vi "Temp - Create DAQ Tasks.vi"(8 "error in (no error)":errorcluster, 10 "DAQ Configuration":T18={"AI Configuration"=[], "AO Configuration"=[], "AI Buffer Size (S)"=10, "sample mode"=10178, "input terminal configuration"=-1, "output terminal configuration"=-1, "Channels: AO"={"AO amp (V)"=[0.1, 0.09, 0.08, 0.07, 0.06, 0.05, 0.04, 0.03], "AO DC (V)"=[0.0, 0.0, 0.0, 0.0, 0.0, 0.0, 0.0, 0.0], "AO f (Hz)"=[13.0, 13.0, 13.0, 13.0, 13.0, 13.0, 13.0, 13.0], "AO phi (°)"=[0.0, 0.0, 0.0, 0.0, 0.0, 0.0, 0.0, 0.0], "function"=[enum."Sine", enum."Sine", enum."Sine", enum."Sine", enum."Sine", enum."Sine", enum."Sine", enum."Sine"], "I+"=[]}, "Channels: Lockin"={"REF f (Hz)"=[0.4, 0.4], "REF phi (°)"=[0.0, 0.0]}, "sampling info"={"Fs"=0.0, "#s"=0.0}} {"Channels: Lockin"."REF phi (°)" format="%#_3g"; "Channels: AO"."AO f (Hz)" min=0.001 max=10000.0; "Channels: AO"."AO DC (V)" format="%.3p"; "Channels: AO"."AO amp (V)" format="%.3p"; "output terminal configuration" items=["Default"=-1, "RSE"=10083, "Differential"=10106, "Pseudodifferential"=12529]; "input terminal configuration" items=["default"=-1, "RSE"=10083, "NRSE"=10078, "Differential"=10106, "Pseudodifferential"=12529]; "sample mode" items=["Finite Samples"=10178, "Continuous Samples"=10123]}, 11 "LockinDAQ in":refnum<class "LockinDAQ.lvclass">) -> (0 "error out":errorcluster, 3 "LockinDAQ out":refnum<class "LockinDAQ.lvclass">)   [LabVIEW 2016, in "LockinDAQ.lvclass"]
uses:
  LockinDAQ.lvclass
  Typedefs/AI.config-array.ctl
  Typedefs/AI.config-cluster.ctl
  Typedefs/AI.coupling-enum.ctl
  Typedefs/446xAI-enum.ctl
  Typedefs/AO.config-array.ctl
  Typedefs/AO.config-cluster.ctl
  Typedefs/446xAO-enum.ctl
  Typedefs/AO-cluster.ctl
  Typedefs/AO_Amp-array.ctl
  Typedefs/AO_DC-array.ctl
  Typedefs/AO_f-array.ctl
  Typedefs/AO_phi-array.ctl
  Typedefs/Function-array.ctl
  Typedefs/Function-enum.ctl
  Typedefs/REF-cluster.ctl
  Typedefs/REF_f-array.ctl
  Typedefs/REF_phi-array.ctl
  LockinDAQ.lvclass/LockinDAQ.ctl
  <vilib>/DAQmx/write.llb/DAQmx Write (Analog 1D Wfm NChan NSamp).vi
  <vilib>/DAQmx/read.llb/DAQmx Read (Analog 1D Wfm NChan NSamp).vi
  <vilib>/DAQmx/create/channels.llb/DAQmx Create Channel (AO-Voltage-Basic).vi
  <vilib>/DAQmx/create/channels.llb/DAQmx Create Channel (AI-Voltage-Basic).vi
  <vilib>/DAQmx/configure/timing.llb/DAQmx Timing (Sample Clock).vi
  <vilib>/DAQmx/configure/trigger.llb/DAQmx Start Trigger (Digital Edge).vi
  <vilib>/DAQmx/miscellaneous.llb/DAQmx Fill In Error Info.vi
  <resource>/objmgr/daqmx.rc
panel:
  out "AI.FilterDelay":dbl
  out "AI.Gain":dbl
  out "SampClk.Timebase.Rate":dbl
  out "SampQuant.SampPerChan":dbl
  # "1"
  # "2"
  # "3"
  # "4"
  # "5"
  # "6"
  # "7"
  # "8"
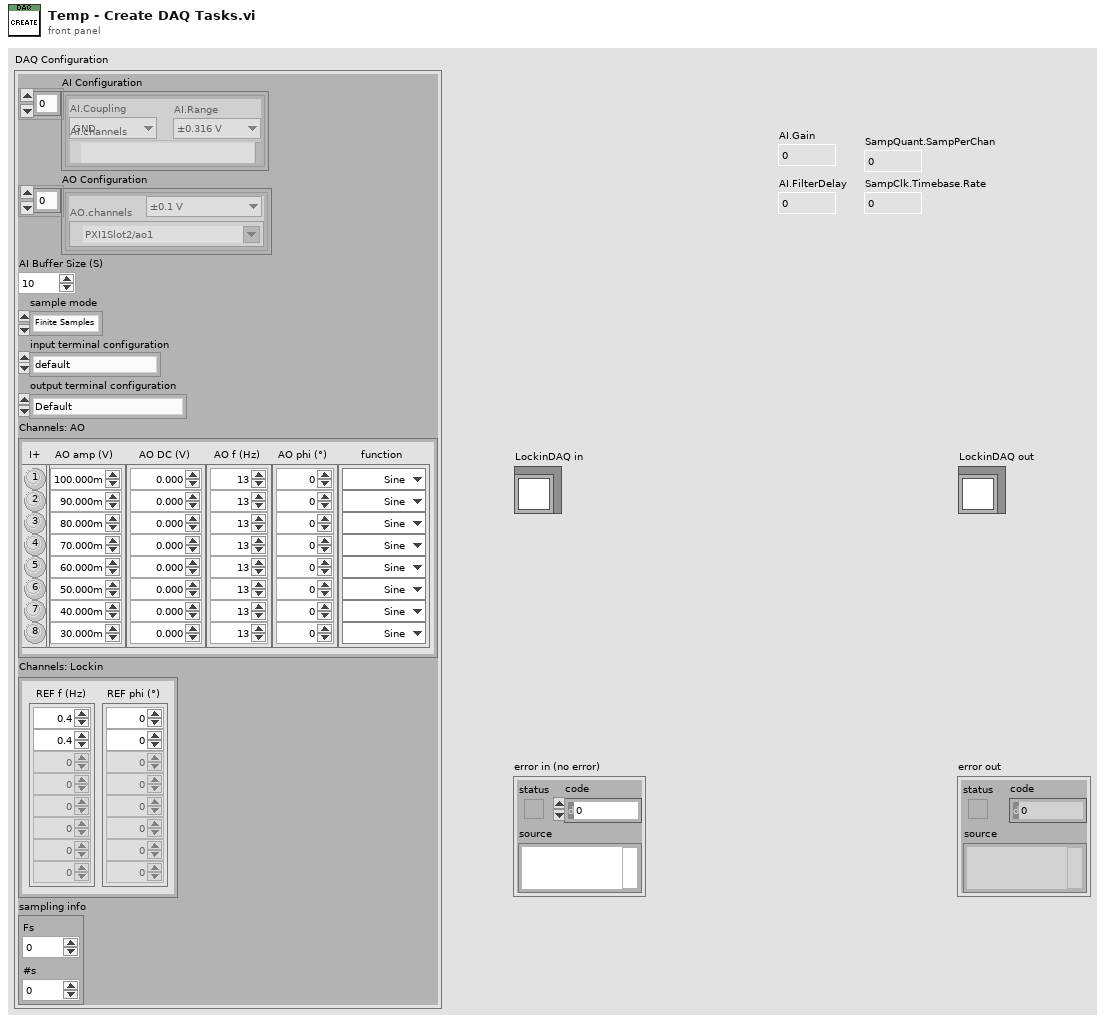
[diagram p1: front panel]
types:
  T1 = typedef "AI.config-array.ctl" = T2[]
  T2 = typedef "AI.config-cluster.ctl" = cluster{"AI.Coupling":T3, "AI.channels":tag, "AI.Range":T4}
  T3 = typedef "AI.coupling-enum.ctl" = enum16{"AC", "DC", "GND"}
  T4 = typedef "446xAI-enum.ctl" = enum16{"±0.316 V", "±1.00 V", "±3.16 V", "±10.0 V", "±31.6 V", "±42.4 V"}
  T5 = typedef "AO.config-array.ctl" = T6[]
  T6 = typedef "AO.config-cluster.ctl" = cluster{"AO.Range":T7, "AO.channels":tag}
  T7 = typedef "446xAO-enum.ctl" = enum16{"±0.1 V", "±1.0 V", "±10.0 V"}
  T8 = typedef "AO-cluster.ctl" = cluster{"AO amp (V)":T9, "AO DC (V)":T10, "AO f (Hz)":T11, "AO phi (°)":T12, "function":T13, "I+":bool[]}
  T9 = typedef "AO_Amp-array.ctl" = dbl[]
  T10 = typedef "AO_DC-array.ctl" = dbl[]
  T11 = typedef "AO_f-array.ctl" = dbl[]
  T12 = typedef "AO_phi-array.ctl" = dbl[]
  T13 = typedef "Function-array.ctl" = T14[]
  T14 = typedef "Function-enum.ctl" = enum16{"Sine", "Triangle", "Square", "Sawtooth"}
  T15 = typedef "REF-cluster.ctl" = cluster{"REF f (Hz)":T16, "REF phi (°)":T17}
  T16 = typedef "REF_f-array.ctl" = dbl[]
  T17 = typedef "REF_phi-array.ctl" = dbl[]
  T18 = cluster{"AI Configuration":T1, "AO Configuration":T5, "AI Buffer Size (S)":i32, "sample mode":i32, "input terminal configuration":i32, "output terminal configuration":i32, "Channels: AO":T8, "Channels: Lockin":T15, "sampling info":cluster{"Fs":dbl, "#s":dbl}}
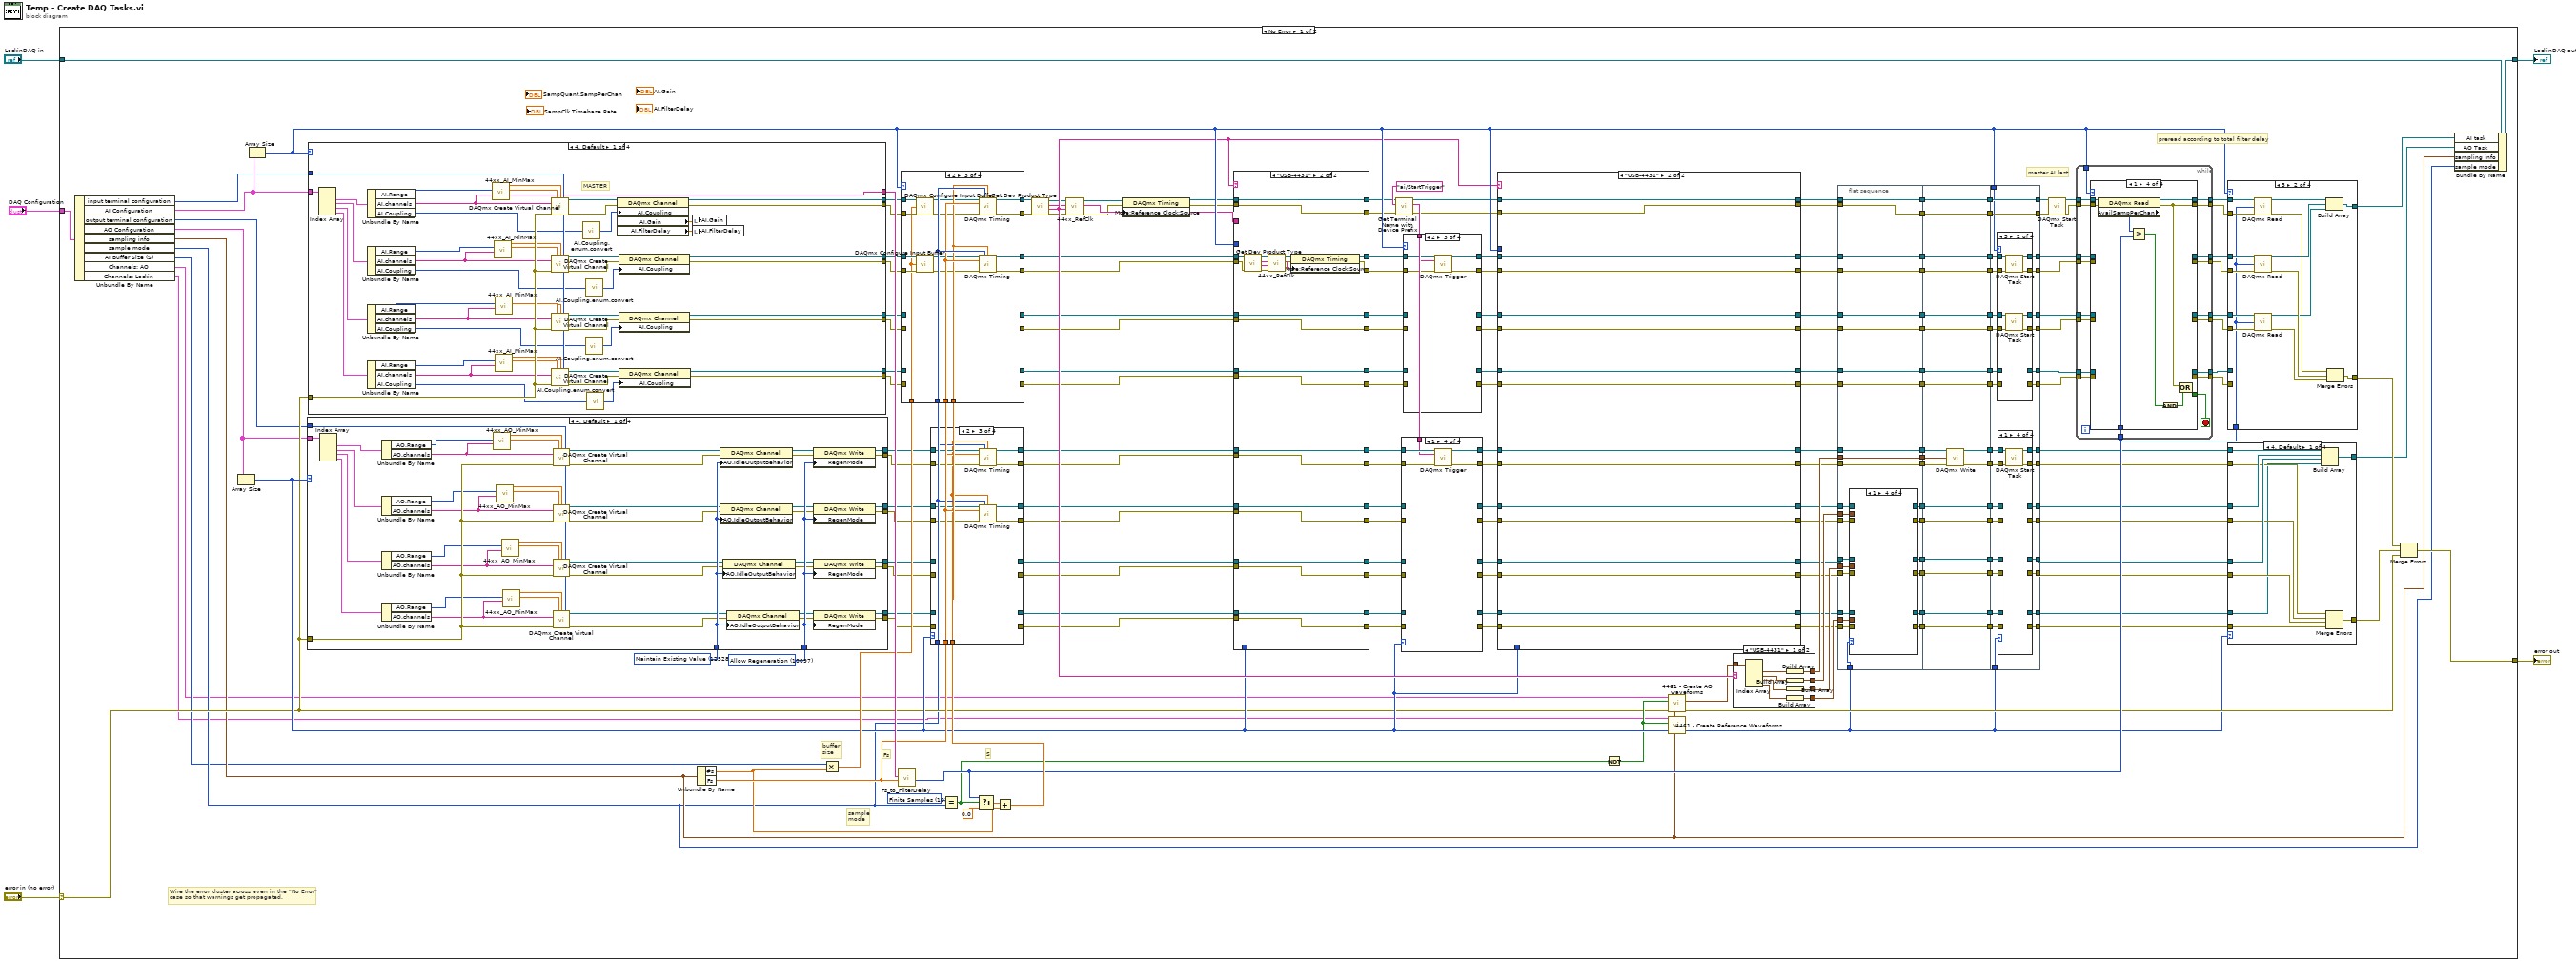
[diagram p0: block diagram]
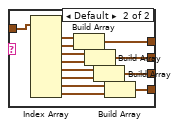
[diagram p2: hidden frame]
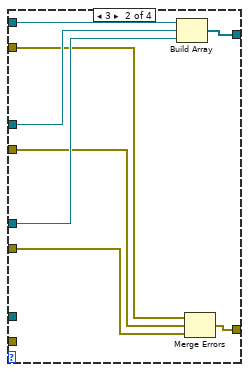
[diagram p3: hidden frame]
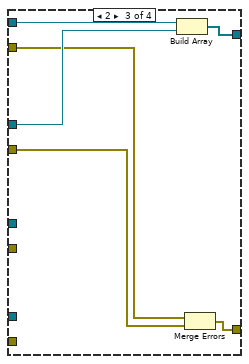
[diagram p4: hidden frame]
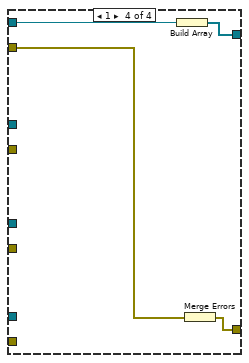
[diagram p5: hidden frame]
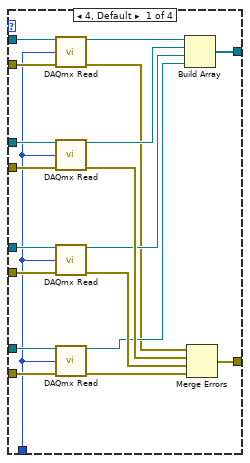
[diagram p6: hidden frame]
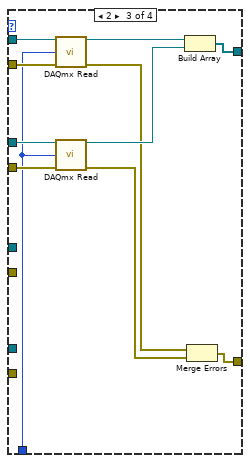
[diagram p7: hidden frame]
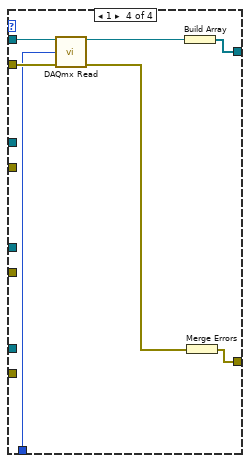
[diagram p8: hidden frame]
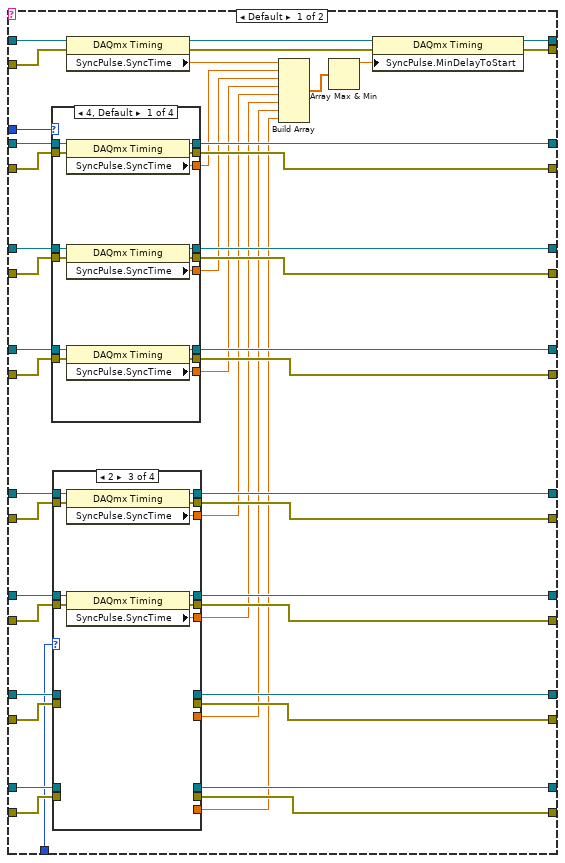
[diagram p9: hidden frame]
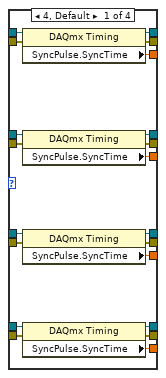
[diagram p10: hidden frame]
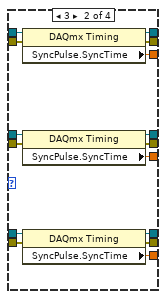
[diagram p11: hidden frame]
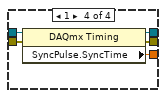
[diagram p12: hidden frame]
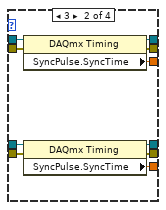
[diagram p13: hidden frame]
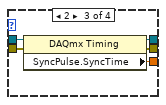
[diagram p14: hidden frame]
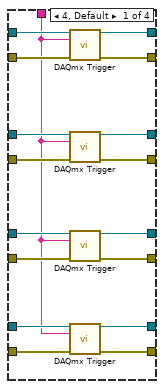
[diagram p16: hidden frame]
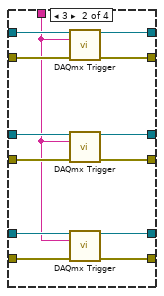
[diagram p17: hidden frame]
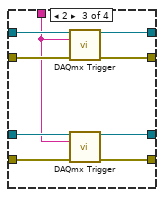
[diagram p18: hidden frame]
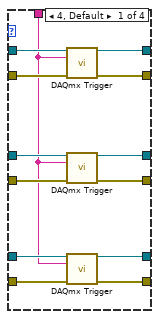
[diagram p19: hidden frame]
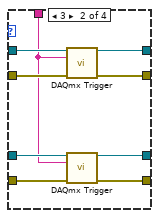
[diagram p20: hidden frame]
diagram:
  n1 = case shown="No Error" "error in (no error)" {
    selector: "error in (no error)" -> [w20 w1306]
    tunnel: [w21 w1306] -> w4
    tunnel: [w18 w1305] -> w2
    tunnel: "LockinDAQ in" -> [w19 w1305]
    tunnel: "DAQ Configuration" -> [w6 _]
    frame No Error {
      w27 = 10097 items=["Allow Regeneration"=10097, "Do Not Allow Regeneration"=10158] ("RegenMode")
      w25 = 12528 items=["Zero Volts"=12526, "High-Impedance"=12527, "Maintain Existing Value"=12528] ("AO.IdleOutputBehavior")
      w24 = 10178 items=["Finite Samples"=10178, "Continuous Samples"=10123] ("sample mode 2")
      # "preread according to total filter delay"
      # "master AI last"
      # "S"
      # "Fs"
      # "sample\nmode"
      # "buffer\nsize"
      # "Wire the error cluster across even in the \"No Error\"\ncase so that warnings get propagated."
      n2 = Unbundle By Name(w6) -> ("input terminal configuration"=w14:i32, "AI Configuration"=w15:T1, "output terminal configuration"=w13:i32, "AO Configuration"=w7:T5, "sampling info"=w12:cluster{"Fs":dbl, "#s":dbl}, "sample mode"=w11:i32, "AI Buffer Size (S)"=w10:i32, "Channels: AO"=w9:T8, "Channels: Lockin"=w8:T15)
      n3 = Array Size(array=w7) -> (size(s)=w30:i32)
      n4 = Array Size(array=w15) -> (size(s)=w157:i32)
      n5 = case shown="4, Default" w30 {
        tunnel: w7 -> [w826 w864 w891 w907]
        tunnel: w20 -> [w794 w839 w873 w896]
        tunnel: w13 -> [w821 w860 w888 w905]
        tunnel: [w816 w855 w883 w900] -> w84
        tunnel: [w815 _ _ _] -> w85
        tunnel: [w814 w854 w882 _] -> w86
        tunnel: [w813 w853 _ _] -> w87
        tunnel: w25 -> [w812 w852 w881 w899]
        tunnel: [w811 w851 w880 w898] -> w96
        tunnel: [w810 w850 w879 _] -> w97
        tunnel: [w809 w849 _ _] -> w98
        tunnel: [w808 _ _ _] -> w99
        tunnel: w27 -> [w807 w848 w878 w897]
        frame 4, Default {
          n6 = Index Array(array=w826) -> (element #1=w825:T6, element #2=w822:T6, element #3=w823:T6, element #4=w824:T6)  [unwired: 4 in]
          n7 = Unbundle By Name(w825) -> ("AO.Range"=w793:T7, "AO.channels"=w781:tag)
          n8 = Unbundle By Name(w822) -> ("AO.Range"=w788:T7, "AO.channels"=w780:tag)
          n9 = Unbundle By Name(w823) -> ("AO.Range"=w789:T7, "AO.channels"=w779:tag)
          n10 = Unbundle By Name(w824) -> ("AO.Range"=w790:T7, "AO.channels"=w778:tag)
          n11 = call "44xx_AO_MinMax.vi"("AO.channels"=w781, "AO.Range"=w793) -> ("AO.max"=w792:dbl, "AO.min"=w791:dbl)  [unwired: 7 in, 1 out]
          n12 = call "44xx_AO_MinMax.vi"("AO.channels"=w780, "AO.Range"=w788) -> ("AO.max"=w787:dbl, "AO.min"=w786:dbl)  [unwired: 7 in, 1 out]
          n13 = call "44xx_AO_MinMax.vi"("AO.channels"=w779, "AO.Range"=w789) -> ("AO.max"=w785:dbl, "AO.min"=w784:dbl)  [unwired: 7 in, 1 out]
          n14 = call "44xx_AO_MinMax.vi"("AO.channels"=w778, "AO.Range"=w790) -> ("AO.max"=w783:dbl, "AO.min"=w782:dbl)  [unwired: 7 in, 1 out]
          n15 = call-poly <vilib>:"DAQmx Create Virtual Channel.vi"("maximum value"=w792, "minimum value"=w791, "output terminal configuration"=w821, "physical channels"=w781, "error in"=w794) -> ("task out"=w820:refnum<k21>, "error out"=w819:errorcluster)  [unwired: 9 in]
          n16 = call-poly <vilib>:"DAQmx Create Virtual Channel.vi"("maximum value"=w787, "minimum value"=w786, "output terminal configuration"=w821, "physical channels"=w780, "error in"=w794) -> ("task out"=w801:refnum<k21>, "error out"=w802:errorcluster)  [unwired: 9 in]
          n17 = call-poly <vilib>:"DAQmx Create Virtual Channel.vi"("maximum value"=w785, "minimum value"=w784, "output terminal configuration"=w821, "physical channels"=w779, "error in"=w794) -> ("task out"=w803:refnum<k21>, "error out"=w804:errorcluster)  [unwired: 9 in]
          n18 = call-poly <vilib>:"DAQmx Create Virtual Channel.vi"("maximum value"=w783, "minimum value"=w782, "output terminal configuration"=w821, "physical channels"=w778, "error in"=w794) -> ("task out"=w806:refnum<k21>, "error out"=w805:errorcluster)  [unwired: 9 in]
          n19 = property class="DAQmx Channel"(reference=w820, error in=w819, "AO.IdleOutputBehavior"=w812) -> (reference out=w818:refnum<k21>, error out=w817:errorcluster)
          n20 = property class="DAQmx Channel"(reference=w801, error in=w802, "AO.IdleOutputBehavior"=w812) -> (reference out=w795:refnum<k21>, error out=w796:errorcluster)
          n21 = property class="DAQmx Channel"(reference=w803, error in=w804, "AO.IdleOutputBehavior"=w812) -> (reference out=w797:refnum<k21>, error out=w798:errorcluster)
          n22 = property class="DAQmx Channel"(reference=w806, error in=w805, "AO.IdleOutputBehavior"=w812) -> (reference out=w800:refnum<k21>, error out=w799:errorcluster)
          n23 = property class="DAQmx Write"(reference=w818, error in=w817, "RegenMode"=w807) -> (reference out=w816:refnum<k21>, error out=w811:errorcluster)
          n24 = property class="DAQmx Write"(reference=w795, error in=w796, "RegenMode"=w807) -> (reference out=w814:refnum<k21>, error out=w810:errorcluster)
          n25 = property class="DAQmx Write"(reference=w797, error in=w798, "RegenMode"=w807) -> (reference out=w813:refnum<k21>, error out=w809:errorcluster)
          n26 = property class="DAQmx Write"(reference=w800, error in=w799, "RegenMode"=w807) -> (reference out=w815:refnum<k21>, error out=w808:errorcluster)
        }
        frame 3 {
          n27 = Index Array(array=w864) -> (element #1=w863:T6, element #2=w861:T6, element #3=w862:T6)  [unwired: 4 in, 1 out]
          n28 = Unbundle By Name(w863) -> ("AO.Range"=w838:T7, "AO.channels"=w827:tag)
          n29 = Unbundle By Name(w861) -> ("AO.Range"=w834:T7, "AO.channels"=w828:tag)
          n30 = Unbundle By Name(w862) -> ("AO.Range"=w835:T7, "AO.channels"=w829:tag)
          n31 = call "44xx_AO_MinMax.vi"("AO.channels"=w827, "AO.Range"=w838) -> ("AO.max"=w837:dbl, "AO.min"=w836:dbl)  [unwired: 7 in, 1 out]
          n32 = call "44xx_AO_MinMax.vi"("AO.channels"=w828, "AO.Range"=w834) -> ("AO.max"=w833:dbl, "AO.min"=w832:dbl)  [unwired: 7 in, 1 out]
          n33 = call "44xx_AO_MinMax.vi"("AO.channels"=w829, "AO.Range"=w835) -> ("AO.max"=w831:dbl, "AO.min"=w830:dbl)  [unwired: 7 in, 1 out]
          n34 = call-poly <vilib>:"DAQmx Create Virtual Channel.vi"("maximum value"=w837, "minimum value"=w836, "output terminal configuration"=w860, "physical channels"=w827, "error in"=w839) -> ("task out"=w859:refnum<k21>, "error out"=w858:errorcluster)  [unwired: 9 in]
          n35 = call-poly <vilib>:"DAQmx Create Virtual Channel.vi"("maximum value"=w833, "minimum value"=w832, "output terminal configuration"=w860, "physical channels"=w828, "error in"=w839) -> ("task out"=w844:refnum<k21>, "error out"=w845:errorcluster)  [unwired: 9 in]
          n36 = call-poly <vilib>:"DAQmx Create Virtual Channel.vi"("maximum value"=w831, "minimum value"=w830, "output terminal configuration"=w860, "physical channels"=w829, "error in"=w839) -> ("task out"=w846:refnum<k21>, "error out"=w847:errorcluster)  [unwired: 9 in]
          n37 = property class="DAQmx Channel"(reference=w859, error in=w858, "AO.IdleOutputBehavior"=w852) -> (reference out=w857:refnum<k21>, error out=w856:errorcluster)
          n38 = property class="DAQmx Channel"(reference=w844, error in=w845, "AO.IdleOutputBehavior"=w852) -> (reference out=w840:refnum<k21>, error out=w841:errorcluster)
          n39 = property class="DAQmx Channel"(reference=w846, error in=w847, "AO.IdleOutputBehavior"=w852) -> (reference out=w842:refnum<k21>, error out=w843:errorcluster)
          n40 = property class="DAQmx Write"(reference=w857, error in=w856, "RegenMode"=w848) -> (reference out=w855:refnum<k21>, error out=w851:errorcluster)
          n41 = property class="DAQmx Write"(reference=w840, error in=w841, "RegenMode"=w848) -> (reference out=w854:refnum<k21>, error out=w850:errorcluster)
          n42 = property class="DAQmx Write"(reference=w842, error in=w843, "RegenMode"=w848) -> (reference out=w853:refnum<k21>, error out=w849:errorcluster)
        }
        frame 2 {
          n43 = Index Array(array=w891) -> (element #1=w890:T6, element #2=w889:T6)  [unwired: 4 in, 2 out]
          n44 = Unbundle By Name(w890) -> ("AO.Range"=w872:T7, "AO.channels"=w866:tag)
          n45 = Unbundle By Name(w889) -> ("AO.Range"=w869:T7, "AO.channels"=w865:tag)
          n46 = call "44xx_AO_MinMax.vi"("AO.channels"=w866, "AO.Range"=w872) -> ("AO.max"=w871:dbl, "AO.min"=w870:dbl)  [unwired: 7 in, 1 out]
          n47 = call "44xx_AO_MinMax.vi"("AO.channels"=w865, "AO.Range"=w869) -> ("AO.max"=w868:dbl, "AO.min"=w867:dbl)  [unwired: 7 in, 1 out]
          n48 = call-poly <vilib>:"DAQmx Create Virtual Channel.vi"("maximum value"=w871, "minimum value"=w870, "output terminal configuration"=w888, "physical channels"=w866, "error in"=w873) -> ("task out"=w887:refnum<k21>, "error out"=w886:errorcluster)  [unwired: 9 in]
          n49 = call-poly <vilib>:"DAQmx Create Virtual Channel.vi"("maximum value"=w868, "minimum value"=w867, "output terminal configuration"=w888, "physical channels"=w865, "error in"=w873) -> ("task out"=w876:refnum<k21>, "error out"=w877:errorcluster)  [unwired: 9 in]
          n50 = property class="DAQmx Channel"(reference=w887, error in=w886, "AO.IdleOutputBehavior"=w881) -> (reference out=w885:refnum<k21>, error out=w884:errorcluster)
          n51 = property class="DAQmx Channel"(reference=w876, error in=w877, "AO.IdleOutputBehavior"=w881) -> (reference out=w874:refnum<k21>, error out=w875:errorcluster)
          n52 = property class="DAQmx Write"(reference=w885, error in=w884, "RegenMode"=w878) -> (reference out=w883:refnum<k21>, error out=w880:errorcluster)
          n53 = property class="DAQmx Write"(reference=w874, error in=w875, "RegenMode"=w878) -> (reference out=w882:refnum<k21>, error out=w879:errorcluster)
        }
        frame 1 {
          n54 = Index Array(array=w907) -> (element #1=w906:T6)  [unwired: 4 in, 3 out]
          n55 = Unbundle By Name(w906) -> ("AO.Range"=w893:T7, "AO.channels"=w892:tag)
          n56 = call "44xx_AO_MinMax.vi"("AO.channels"=w892, "AO.Range"=w893) -> ("AO.max"=w895:dbl, "AO.min"=w894:dbl)  [unwired: 7 in, 1 out]
          n57 = call-poly <vilib>:"DAQmx Create Virtual Channel.vi"("maximum value"=w895, "minimum value"=w894, "output terminal configuration"=w905, "physical channels"=w892, "error in"=w896) -> ("task out"=w904:refnum<k21>, "error out"=w903:errorcluster)  [unwired: 9 in]
          n58 = property class="DAQmx Channel"(reference=w904, error in=w903, "AO.IdleOutputBehavior"=w899) -> (reference out=w902:refnum<k21>, error out=w901:errorcluster)
          n59 = property class="DAQmx Write"(reference=w902, error in=w901, "RegenMode"=w897) -> (reference out=w900:refnum<k21>, error out=w898:errorcluster)
        }
      }
      n60 = case shown="4, Default" w157 {
        tunnel: w15 -> [w957 w996 w1024 w1041]
        tunnel: w20 -> [w956 w995 w1023 w1040]
        tunnel: w14 -> [w955 w994 w1022 w1039]
        tunnel: [w954 w993 w1021 _] -> w93
        tunnel: [w953 w992 _ _] -> w94
        tunnel: [w952 _ _ _] -> w95
        tunnel: [w951 w991 w1020 _] -> w145
        tunnel: [w950 w990 _ _] -> w146
        tunnel: [w949 _ _ _] -> w147
        tunnel: [w948 w989 w1019 w1038] -> w120
        tunnel: [w947 w988 w1018 w1037] -> w144
        tunnel: [w908 w958 w997 w1025] -> w161
        frame 4, Default {
          # "MASTER"
          n61 = Index Array(array=w957) -> (element #1=w922:T2, element #2=w944:T2, element #3=w943:T2, element #4=w942:T2)  [unwired: 4 in]
          n62 = Unbundle By Name(w922) -> ("AI.Range"=w923:T4, "AI.channels"=w914:tag, "AI.Coupling"=w939:T3)
          n63 = Unbundle By Name(w944) -> ("AI.Range"=w912:T4, "AI.channels"=w913:tag, "AI.Coupling"=w930:T3)
          n64 = Unbundle By Name(w943) -> ("AI.Range"=w921:T4, "AI.channels"=w911:tag, "AI.Coupling"=w931:T3)
          n65 = Unbundle By Name(w942) -> ("AI.Range"=w910:T4, "AI.channels"=w909:tag, "AI.Coupling"=w932:T3)
          n66 = call "44xx_AI_MinMax.vi"("AI.channels"=w914, "446x AI"=w923) -> ("ProductType"=w908:string, "AI.Max"=w925:dbl, "AI.Min"=w924:dbl)  [unwired: 7 in]
          n67 = call "44xx_AI_MinMax.vi"("AI.channels"=w913, "446x AI"=w912) -> ("AI.Max"=w920:dbl, "AI.Min"=w917:dbl)  [unwired: 7 in, 1 out]
          n68 = call "44xx_AI_MinMax.vi"("AI.channels"=w909, "446x AI"=w910) -> ("AI.Max"=w916:dbl, "AI.Min"=w915:dbl)  [unwired: 7 in, 1 out]
          n69 = call "44xx_AI_MinMax.vi"("AI.channels"=w911, "446x AI"=w921) -> ("AI.Max"=w919:dbl, "AI.Min"=w918:dbl)  [unwired: 7 in, 1 out]
          n70 = call-poly <vilib>:"DAQmx Create Virtual Channel.vi"("maximum value"=w925, "minimum value"=w924, "input terminal configuration"=w955, "physical channels"=w914, "error in"=w956) -> ("task out"=w946:refnum<k21>, "error out"=w945:errorcluster)  [unwired: 9 in]
          n71 = call-poly <vilib>:"DAQmx Create Virtual Channel.vi"("maximum value"=w920, "minimum value"=w917, "input terminal configuration"=w955, "physical channels"=w913, "error in"=w956) -> ("task out"=w937:refnum<k21>, "error out"=w938:errorcluster)  [unwired: 9 in]
          n72 = call-poly <vilib>:"DAQmx Create Virtual Channel.vi"("maximum value"=w919, "minimum value"=w918, "input terminal configuration"=w955, "physical channels"=w911, "error in"=w956) -> ("task out"=w936:refnum<k21>, "error out"=w935:errorcluster)  [unwired: 9 in]
          n73 = call-poly <vilib>:"DAQmx Create Virtual Channel.vi"("maximum value"=w916, "minimum value"=w915, "input terminal configuration"=w955, "physical channels"=w909, "error in"=w956) -> ("task out"=w933:refnum<k21>, "error out"=w934:errorcluster)  [unwired: 9 in]
          n74 = call "AI.Coupling.enum.convert.vi"("AI.Coupling"=w939) -> ("Numeric"=w929:i32)
          n75 = call "AI.Coupling.enum.convert.vi"("AI.Coupling"=w931) -> ("Numeric"=w927:i32)
          n76 = call "AI.Coupling.enum.convert.vi"("AI.Coupling"=w930) -> ("Numeric"=w928:i32)
          n77 = call "AI.Coupling.enum.convert.vi"("AI.Coupling"=w932) -> ("Numeric"=w926:i32)
          n78 = property class="DAQmx Channel"(reference=w946, error in=w945, "AI.Coupling"=w929) -> (reference out=w948:refnum<k21>, error out=w947:errorcluster, "AI.Gain"=w941:dbl, "AI.FilterDelay"=w940:dbl)
          n79 = property class="DAQmx Channel"(reference=w937, error in=w938, "AI.Coupling"=w928) -> (reference out=w954:refnum<k21>, error out=w951:errorcluster)
          n80 = property class="DAQmx Channel"(reference=w936, error in=w935, "AI.Coupling"=w927) -> (reference out=w953:refnum<k21>, error out=w950:errorcluster)
          n81 = property class="DAQmx Channel"(reference=w933, error in=w934, "AI.Coupling"=w926) -> (reference out=w952:refnum<k21>, error out=w949:errorcluster)
          n82 = local write "AI.Gain"(w941) -> ()
          n83 = local write "AI.FilterDelay"(w940) -> ()
        }
        frame 3 {
          # "MASTER"
          n84 = Index Array(array=w996) -> (element #1=w968:T2, element #2=w985:T2, element #3=w984:T2)  [unwired: 4 in, 1 out]
          n85 = Unbundle By Name(w968) -> ("AI.Range"=w969:T4, "AI.channels"=w959:tag, "AI.Coupling"=w981:T3)
          n86 = Unbundle By Name(w985) -> ("AI.Range"=w960:T4, "AI.channels"=w961:tag, "AI.Coupling"=w975:T3)
          n87 = Unbundle By Name(w984) -> ("AI.Range"=w967:T4, "AI.channels"=w962:tag, "AI.Coupling"=w976:T3)
          n88 = call "44xx_AI_MinMax.vi"("AI.channels"=w959, "446x AI"=w969) -> ("ProductType"=w958:string, "AI.Max"=w971:dbl, "AI.Min"=w970:dbl)  [unwired: 7 in]
          n89 = call "44xx_AI_MinMax.vi"("AI.channels"=w961, "446x AI"=w960) -> ("AI.Max"=w966:dbl, "AI.Min"=w963:dbl)  [unwired: 7 in, 1 out]
          n90 = call "44xx_AI_MinMax.vi"("AI.channels"=w962, "446x AI"=w967) -> ("AI.Max"=w965:dbl, "AI.Min"=w964:dbl)  [unwired: 7 in, 1 out]
          n91 = call-poly <vilib>:"DAQmx Create Virtual Channel.vi"("maximum value"=w971, "minimum value"=w970, "input terminal configuration"=w994, "physical channels"=w959, "error in"=w995) -> ("task out"=w987:refnum<k21>, "error out"=w986:errorcluster)  [unwired: 9 in]
          n92 = call-poly <vilib>:"DAQmx Create Virtual Channel.vi"("maximum value"=w966, "minimum value"=w963, "input terminal configuration"=w994, "physical channels"=w961, "error in"=w995) -> ("task out"=w979:refnum<k21>, "error out"=w980:errorcluster)  [unwired: 9 in]
          n93 = call-poly <vilib>:"DAQmx Create Virtual Channel.vi"("maximum value"=w965, "minimum value"=w964, "input terminal configuration"=w994, "physical channels"=w962, "error in"=w995) -> ("task out"=w978:refnum<k21>, "error out"=w977:errorcluster)  [unwired: 9 in]
          n94 = call "AI.Coupling.enum.convert.vi"("AI.Coupling"=w981) -> ("Numeric"=w974:i32)
          n95 = call "AI.Coupling.enum.convert.vi"("AI.Coupling"=w976) -> ("Numeric"=w972:i32)
          n96 = call "AI.Coupling.enum.convert.vi"("AI.Coupling"=w975) -> ("Numeric"=w973:i32)
          n97 = property class="DAQmx Channel"(reference=w987, error in=w986, "AI.Coupling"=w974) -> (reference out=w989:refnum<k21>, error out=w988:errorcluster, "AI.Gain"=w983:dbl, "AI.FilterDelay"=w982:dbl)
          n98 = property class="DAQmx Channel"(reference=w979, error in=w980, "AI.Coupling"=w973) -> (reference out=w993:refnum<k21>, error out=w991:errorcluster)
          n99 = property class="DAQmx Channel"(reference=w978, error in=w977, "AI.Coupling"=w972) -> (reference out=w992:refnum<k21>, error out=w990:errorcluster)
          n100 = local write "AI.Gain"(w983) -> ()
          n101 = local write "AI.FilterDelay"(w982) -> ()
        }
        frame 2 {
          # "MASTER"
          n102 = Index Array(array=w1024) -> (element #1=w1003:T2, element #2=w1015:T2)  [unwired: 4 in, 2 out]
          n103 = Unbundle By Name(w1003) -> ("AI.Range"=w1004:T4, "AI.channels"=w998:tag, "AI.Coupling"=w1012:T3)
          n104 = Unbundle By Name(w1015) -> ("AI.Range"=w1000:T4, "AI.channels"=w999:tag, "AI.Coupling"=w1009:T3)
          n105 = call "44xx_AI_MinMax.vi"("AI.channels"=w998, "446x AI"=w1004) -> ("ProductType"=w997:string, "AI.Max"=w1006:dbl, "AI.Min"=w1005:dbl)  [unwired: 7 in]
          n106 = call "44xx_AI_MinMax.vi"("AI.channels"=w999, "446x AI"=w1000) -> ("AI.Max"=w1002:dbl, "AI.Min"=w1001:dbl)  [unwired: 7 in, 1 out]
          n107 = call-poly <vilib>:"DAQmx Create Virtual Channel.vi"("maximum value"=w1006, "minimum value"=w1005, "input terminal configuration"=w1022, "physical channels"=w998, "error in"=w1023) -> ("task out"=w1017:refnum<k21>, "error out"=w1016:errorcluster)  [unwired: 9 in]
          n108 = call-poly <vilib>:"DAQmx Create Virtual Channel.vi"("maximum value"=w1002, "minimum value"=w1001, "input terminal configuration"=w1022, "physical channels"=w999, "error in"=w1023) -> ("task out"=w1010:refnum<k21>, "error out"=w1011:errorcluster)  [unwired: 9 in]
          n109 = call "AI.Coupling.enum.convert.vi"("AI.Coupling"=w1012) -> ("Numeric"=w1008:i32)
          n110 = call "AI.Coupling.enum.convert.vi"("AI.Coupling"=w1009) -> ("Numeric"=w1007:i32)
          n111 = property class="DAQmx Channel"(reference=w1017, error in=w1016, "AI.Coupling"=w1008) -> (reference out=w1019:refnum<k21>, error out=w1018:errorcluster, "AI.Gain"=w1014:dbl, "AI.FilterDelay"=w1013:dbl)
          n112 = property class="DAQmx Channel"(reference=w1010, error in=w1011, "AI.Coupling"=w1007) -> (reference out=w1021:refnum<k21>, error out=w1020:errorcluster)
          n113 = local write "AI.Gain"(w1014) -> ()
          n114 = local write "AI.FilterDelay"(w1013) -> ()
        }
        frame 1 {
          # "MASTER"
          n115 = Index Array(array=w1041) -> (element #1=w1030:T2)  [unwired: 4 in, 3 out]
          n116 = Unbundle By Name(w1030) -> ("AI.Range"=w1029:T4, "AI.channels"=w1028:tag, "AI.Coupling"=w1032:T3)
          n117 = call "44xx_AI_MinMax.vi"("AI.channels"=w1028, "446x AI"=w1029) -> ("ProductType"=w1025:string, "AI.Max"=w1027:dbl, "AI.Min"=w1026:dbl)  [unwired: 7 in]
          n118 = call-poly <vilib>:"DAQmx Create Virtual Channel.vi"("maximum value"=w1027, "minimum value"=w1026, "input terminal configuration"=w1039, "physical channels"=w1028, "error in"=w1040) -> ("task out"=w1036:refnum<k21>, "error out"=w1035:errorcluster)  [unwired: 9 in]
          n119 = call "AI.Coupling.enum.convert.vi"("AI.Coupling"=w1032) -> ("Numeric"=w1031:i32)
          n120 = property class="DAQmx Channel"(reference=w1036, error in=w1035, "AI.Coupling"=w1031) -> (reference out=w1038:refnum<k21>, error out=w1037:errorcluster, "AI.Gain"=w1034:dbl, "AI.FilterDelay"=w1033:dbl)
          n121 = local write "AI.Gain"(w1034) -> ()
          n122 = local write "AI.FilterDelay"(w1033) -> ()
        }
      }
      n123 = Unbundle By Name(w12) -> ("#s"=w26:dbl, "Fs"=w158:dbl)
      n124 = Multiply(x=w10, y=w26) -> (x*y=w143:dbl)
      n125 = call "Fs_to_FilterDelay.vi"("Fs"=w158, "ProductType"=w161) -> ("Total Filter Delay (samples)"=w159:u32)  [unwired: 9 in]
      n126 = Equal?(x=w24, y=w11) -> (x = y?=w28:bool)
      n127 = Select(t=w159, s=w28, f=0.0) -> (s? t:f=w23:dbl)
      n128 = Add(x=w23, y=w26) -> (x+y=w160:dbl)
      n129 = case shown="2" w157 {
        tunnel: [w729 w751 w767 w777] -> w149
        tunnel: [w728 w750 w766 w776] -> w148
        tunnel: [w727 w749 w765 _] -> w37
        tunnel: [w726 w748 w764 _] -> w38
        tunnel: [w725 w747 _ _] -> w43
        tunnel: [w724 w746 _ _] -> w44
        tunnel: [w723 _ _ _] -> w45
        tunnel: [w722 _ _ _] -> w46
        tunnel: w95 -> [w712 _ _ _]
        tunnel: w94 -> [w714 w738 _ _]
        tunnel: w146 -> [w707 w735 _ _]
        tunnel: w147 -> [w713 _ _ _]
        tunnel: w145 -> [w716 w740 w758 _]
        tunnel: w93 -> [w715 w739 w757 _]
        tunnel: w11 -> [w721 w745 w763 w775]
        tunnel: w158 -> [w720 w744 w762 w774]
        tunnel: w160 -> [w719 w743 w761 w773]
        tunnel: w144 -> [w718 w742 w760 w772]
        tunnel: w120 -> [w717 w741 w759 w771]
        tunnel: w143 -> [w702 w730 w752 w768]
        frame 4, Default {
          n130 = call <vilib>:"DAQmx Configure Input Buffer.vi"("task/channels in"=w717, "buffer size (in samples per channel)"=w702, "error in"=w718) -> ("task out"=w703:refnum<k21>, "error out"=w704:errorcluster)  [unwired: 11 in]
          n131 = call <vilib>:"DAQmx Configure Input Buffer.vi"("task/channels in"=w715, "buffer size (in samples per channel)"=w702, "error in"=w716) -> ("task out"=w705:refnum<k21>, "error out"=w706:errorcluster)  [unwired: 11 in]
          n132 = call <vilib>:"DAQmx Configure Input Buffer.vi"("task/channels in"=w714, "buffer size (in samples per channel)"=w702, "error in"=w707) -> ("task out"=w708:refnum<k21>, "error out"=w709:errorcluster)  [unwired: 11 in]
          n133 = call <vilib>:"DAQmx Configure Input Buffer.vi"("task/channels in"=w712, "buffer size (in samples per channel)"=w702, "error in"=w713) -> ("task out"=w711:refnum<k21>, "error out"=w710:errorcluster)  [unwired: 11 in]
          n134 = call-poly <vilib>:"DAQmx Timing.vi"("task/channels in"=w703, "sample mode"=w721, "samples per channel"=w719, "rate"=w720, "error in"=w704) -> ("task out"=w729:refnum<k21>, "error out"=w728:errorcluster)  [unwired: 9 in]
          n135 = call-poly <vilib>:"DAQmx Timing.vi"("task/channels in"=w705, "sample mode"=w721, "samples per channel"=w719, "rate"=w720, "error in"=w706) -> ("task out"=w727:refnum<k21>, "error out"=w726:errorcluster)  [unwired: 9 in]
          n136 = call-poly <vilib>:"DAQmx Timing.vi"("task/channels in"=w708, "sample mode"=w721, "samples per channel"=w719, "rate"=w720, "error in"=w709) -> ("task out"=w724:refnum<k21>, "error out"=w725:errorcluster)  [unwired: 9 in]
          n137 = call-poly <vilib>:"DAQmx Timing.vi"("task/channels in"=w711, "sample mode"=w721, "samples per channel"=w719, "rate"=w720, "error in"=w710) -> ("task out"=w723:refnum<k21>, "error out"=w722:errorcluster)  [unwired: 9 in]
        }
        frame 3 {
          n138 = call <vilib>:"DAQmx Configure Input Buffer.vi"("task/channels in"=w741, "buffer size (in samples per channel)"=w730, "error in"=w742) -> ("task out"=w731:refnum<k21>, "error out"=w732:errorcluster)  [unwired: 11 in]
          n139 = call <vilib>:"DAQmx Configure Input Buffer.vi"("task/channels in"=w739, "buffer size (in samples per channel)"=w730, "error in"=w740) -> ("task out"=w733:refnum<k21>, "error out"=w734:errorcluster)  [unwired: 11 in]
          n140 = call <vilib>:"DAQmx Configure Input Buffer.vi"("task/channels in"=w738, "buffer size (in samples per channel)"=w730, "error in"=w735) -> ("task out"=w736:refnum<k21>, "error out"=w737:errorcluster)  [unwired: 11 in]
          n141 = call-poly <vilib>:"DAQmx Timing.vi"("task/channels in"=w731, "sample mode"=w745, "samples per channel"=w743, "rate"=w744, "error in"=w732) -> ("task out"=w751:refnum<k21>, "error out"=w750:errorcluster)  [unwired: 9 in]
          n142 = call-poly <vilib>:"DAQmx Timing.vi"("task/channels in"=w733, "sample mode"=w745, "samples per channel"=w743, "rate"=w744, "error in"=w734) -> ("task out"=w749:refnum<k21>, "error out"=w748:errorcluster)  [unwired: 9 in]
          n143 = call-poly <vilib>:"DAQmx Timing.vi"("task/channels in"=w736, "sample mode"=w745, "samples per channel"=w743, "rate"=w744, "error in"=w737) -> ("task out"=w746:refnum<k21>, "error out"=w747:errorcluster)  [unwired: 9 in]
        }
        frame 2 {
          n144 = call <vilib>:"DAQmx Configure Input Buffer.vi"("task/channels in"=w759, "buffer size (in samples per channel)"=w752, "error in"=w760) -> ("task out"=w753:refnum<k21>, "error out"=w754:errorcluster)  [unwired: 11 in]
          n145 = call <vilib>:"DAQmx Configure Input Buffer.vi"("task/channels in"=w757, "buffer size (in samples per channel)"=w752, "error in"=w758) -> ("task out"=w755:refnum<k21>, "error out"=w756:errorcluster)  [unwired: 11 in]
          n146 = call-poly <vilib>:"DAQmx Timing.vi"("task/channels in"=w753, "sample mode"=w763, "samples per channel"=w761, "rate"=w762, "error in"=w754) -> ("task out"=w767:refnum<k21>, "error out"=w766:errorcluster)  [unwired: 9 in]
          n147 = call-poly <vilib>:"DAQmx Timing.vi"("task/channels in"=w755, "sample mode"=w763, "samples per channel"=w761, "rate"=w762, "error in"=w756) -> ("task out"=w765:refnum<k21>, "error out"=w764:errorcluster)  [unwired: 9 in]
        }
        frame 1 {
          n148 = call <vilib>:"DAQmx Configure Input Buffer.vi"("task/channels in"=w771, "buffer size (in samples per channel)"=w768, "error in"=w772) -> ("task out"=w769:refnum<k21>, "error out"=w770:errorcluster)  [unwired: 11 in]
          n149 = call-poly <vilib>:"DAQmx Timing.vi"("task/channels in"=w769, "sample mode"=w775, "samples per channel"=w773, "rate"=w774, "error in"=w770) -> ("task out"=w777:refnum<k21>, "error out"=w776:errorcluster)  [unwired: 9 in]
        }
      }
      n150 = case shown="2" w30 {
        tunnel: w84 -> [w668 w683 w694 w701]
        tunnel: w85 -> [w667 _ _ _]
        tunnel: w86 -> [w666 w682 w693 _]
        tunnel: w87 -> [w665 w681 _ _]
        tunnel: [w664 w680 w692 _] -> w88
        tunnel: [w663 _ _ _] -> w89
        tunnel: [w662 _ _ _] -> w90
        tunnel: [w661 w679 _ _] -> w91
        tunnel: [w660 w678 w691 w700] -> w92
        tunnel: w11 -> [w659 w677 w690 w699]
        tunnel: w158 -> [w658 w676 w689 w698]
        tunnel: w160 -> [w650 w669 w684 w695]
        tunnel: w96 -> [w657 w675 w688 w697]
        tunnel: w97 -> [w656 w674 w687 _]
        tunnel: w98 -> [w655 w673 _ _]
        tunnel: w99 -> [w654 _ _ _]
        tunnel: [w653 w672 w686 w696] -> w136
        tunnel: [w652 w671 w685 _] -> w116
        tunnel: [w651 w670 _ _] -> w117
        frame 4, Default {
          n151 = call-poly <vilib>:"DAQmx Timing.vi"("task/channels in"=w668, "sample mode"=w659, "samples per channel"=w650, "rate"=w658, "error in"=w657) -> ("task out"=w660:refnum<k21>, "error out"=w653:errorcluster)  [unwired: 9 in]
          n152 = call-poly <vilib>:"DAQmx Timing.vi"("task/channels in"=w666, "sample mode"=w659, "samples per channel"=w650, "rate"=w658, "error in"=w656) -> ("task out"=w664:refnum<k21>, "error out"=w652:errorcluster)  [unwired: 9 in]
          n153 = call-poly <vilib>:"DAQmx Timing.vi"("task/channels in"=w665, "sample mode"=w659, "samples per channel"=w650, "rate"=w658, "error in"=w655) -> ("task out"=w661:refnum<k21>, "error out"=w651:errorcluster)  [unwired: 9 in]
          n154 = call-poly <vilib>:"DAQmx Timing.vi"("task/channels in"=w667, "sample mode"=w659, "samples per channel"=w650, "rate"=w658, "error in"=w654) -> ("task out"=w662:refnum<k21>, "error out"=w663:errorcluster)  [unwired: 9 in]
        }
        frame 3 {
          n155 = call-poly <vilib>:"DAQmx Timing.vi"("task/channels in"=w683, "sample mode"=w677, "samples per channel"=w669, "rate"=w676, "error in"=w675) -> ("task out"=w678:refnum<k21>, "error out"=w672:errorcluster)  [unwired: 9 in]
          n156 = call-poly <vilib>:"DAQmx Timing.vi"("task/channels in"=w682, "sample mode"=w677, "samples per channel"=w669, "rate"=w676, "error in"=w674) -> ("task out"=w680:refnum<k21>, "error out"=w671:errorcluster)  [unwired: 9 in]
          n157 = call-poly <vilib>:"DAQmx Timing.vi"("task/channels in"=w681, "sample mode"=w677, "samples per channel"=w669, "rate"=w676, "error in"=w673) -> ("task out"=w679:refnum<k21>, "error out"=w670:errorcluster)  [unwired: 9 in]
        }
        frame 2 {
          n158 = call-poly <vilib>:"DAQmx Timing.vi"("task/channels in"=w694, "sample mode"=w690, "samples per channel"=w684, "rate"=w689, "error in"=w688) -> ("task out"=w691:refnum<k21>, "error out"=w686:errorcluster)  [unwired: 9 in]
          n159 = call-poly <vilib>:"DAQmx Timing.vi"("task/channels in"=w693, "sample mode"=w690, "samples per channel"=w684, "rate"=w689, "error in"=w687) -> ("task out"=w692:refnum<k21>, "error out"=w685:errorcluster)  [unwired: 9 in]
        }
        frame 1 {
          n160 = call-poly <vilib>:"DAQmx Timing.vi"("task/channels in"=w701, "sample mode"=w699, "samples per channel"=w695, "rate"=w698, "error in"=w697) -> ("task out"=w700:refnum<k21>, "error out"=w696:errorcluster)  [unwired: 9 in]
        }
      }
      n161 = call "Get Dev Product Type.vi"("error in (no error)"=w148, "Refnum in"=w149) -> ("error out"=w154:errorcluster, "ProductType"=w155:string, "ActiveDev"=w150:tag, "Refnum out"=w151:refnum<k21>)  [unwired: 6 in]
      n162 = call "44xx_RefClk.vi"("error in (no error)"=w154, "ProductType"=w155, "ActiveDev"=w150, "Refnum in"=w151) -> ("error out"=w153:errorcluster, "RefClk.Src"=w156:tag, "Refnum out"=w152:refnum<k21>)  [unwired: 5 in]
      n163 = property class="DAQmx Timing"(reference=w152, error in=w153, "More:Reference Clock:Source"=w156) -> (reference out=w77:refnum<k21>, error out=w135:errorcluster)
      n164 = case shown="\"USB-4431\"" w155 {
        tunnel: [w546 w649] -> w33
        tunnel: [w545 w648] -> w34
        tunnel: w37 -> [w544 w635]
        tunnel: w38 -> [w543 w631]
        tunnel: [w542 w625] -> w39
        tunnel: [w541 w626] -> w40
        tunnel: [w540 w646] -> w41
        tunnel: [w539 w647] -> w42
        tunnel: w43 -> [w538 w646]
        tunnel: w44 -> [w537 w647]
        tunnel: w45 -> [w536 w645]
        tunnel: w46 -> [w535 w644]
        tunnel: [w534 w645] -> w47
        tunnel: [w533 w644] -> w48
        tunnel: [w532 w643] -> w50
        tunnel: [w531 w642] -> w51
        tunnel: [w530 w640] -> w54
        tunnel: [w529 w641] -> w55
        tunnel: [w528 w639] -> w56
        tunnel: [w527 w638] -> w57
        tunnel: [w526 w636] -> w58
        tunnel: [w525 w637] -> w59
        tunnel: w77 -> [w524 w649]
        tunnel: w88 -> [w523 w641]
        tunnel: w89 -> [w522 w636]
        tunnel: w90 -> [w521 w637]
        tunnel: w91 -> [w520 w639]
        tunnel: w92 -> [w519 w643]
        tunnel: w116 -> [w517 w640]
        tunnel: w117 -> [w516 w638]
        tunnel: w135 -> [w513 w648]
        tunnel: w156 -> [w512 _]
        tunnel: w157 -> [w510 _]
        tunnel: w136 -> [w518 w642]
        tunnel: w30 -> [w511 _]
        frame Default {
          n165 = call "Get Terminal Name with Device Prefix.vi"("error in (no error)"=w513, "Local Terminal Name"="SyncPulse", "task/channels in"=w524) -> ("error out"=w545:errorcluster, "Terminal Name with Device Prefix"=w514:tag, "task out"=w546:refnum<k21>)  [unwired: 6 in]
          n166 = case shown="2" w511 {
            tunnel: [w564 w578 w588 w594] -> w532
            tunnel: [w563 w577 w587 w593] -> w531
            tunnel: [w562 w576 w586 _] -> w530
            tunnel: [w561 w575 w585 _] -> w529
            tunnel: [w560 w574 _ _] -> w528
            tunnel: [w559 w573 _ _] -> w527
            tunnel: [w558 _ _ _] -> w526
            tunnel: [w557 _ _ _] -> w525
            tunnel: w523 -> [w556 w572 w584 _]
            tunnel: w522 -> [w555 _ _ _]
            tunnel: w521 -> [w554 _ _ _]
            tunnel: w520 -> [w553 w571 _ _]
            tunnel: w519 -> [w552 w570 w583 w592]
            tunnel: w518 -> [w551 w569 w582 w591]
            tunnel: w517 -> [w550 w568 w581 _]
            tunnel: w516 -> [w549 w567 _ _]
            tunnel: w514 -> [w548 w566 w580 w590]
            tunnel: w512 -> [w547 w565 w579 w589]
            frame 4, Default {
              n167 = property class="DAQmx Timing"(reference=w552, error in=w551, "More:Reference Clock:Source"=w547, "More:Synchronization Pulse:Source"=w548) -> (reference out=w564:refnum<k21>, error out=w563:errorcluster)
              n168 = property class="DAQmx Timing"(reference=w556, error in=w550, "More:Reference Clock:Source"=w547, "More:Synchronization Pulse:Source"=w548) -> (reference out=w561:refnum<k21>, error out=w562:errorcluster)
              n169 = property class="DAQmx Timing"(reference=w553, error in=w549, "More:Reference Clock:Source"=w547, "More:Synchronization Pulse:Source"=w548) -> (reference out=w560:refnum<k21>, error out=w559:errorcluster)
              n170 = property class="DAQmx Timing"(reference=w554, error in=w555, "More:Reference Clock:Source"=w547, "More:Synchronization Pulse:Source"=w548) -> (reference out=w557:refnum<k21>, error out=w558:errorcluster)
            }
            frame 3 {
              n171 = property class="DAQmx Timing"(reference=w570, error in=w569, "More:Reference Clock:Source"=w565, "More:Synchronization Pulse:Source"=w566) -> (reference out=w578:refnum<k21>, error out=w577:errorcluster)
              n172 = property class="DAQmx Timing"(reference=w572, error in=w568, "More:Reference Clock:Source"=w565, "More:Synchronization Pulse:Source"=w566) -> (reference out=w575:refnum<k21>, error out=w576:errorcluster)
              n173 = property class="DAQmx Timing"(reference=w571, error in=w567, "More:Reference Clock:Source"=w565, "More:Synchronization Pulse:Source"=w566) -> (reference out=w574:refnum<k21>, error out=w573:errorcluster)
            }
            frame 2 {
              n174 = property class="DAQmx Timing"(reference=w583, error in=w582, "More:Reference Clock:Source"=w579, "More:Synchronization Pulse:Source"=w580) -> (reference out=w588:refnum<k21>, error out=w587:errorcluster)
              n175 = property class="DAQmx Timing"(reference=w584, error in=w581, "More:Reference Clock:Source"=w579, "More:Synchronization Pulse:Source"=w580) -> (reference out=w585:refnum<k21>, error out=w586:errorcluster)
            }
            frame 1 {
              n176 = property class="DAQmx Timing"(reference=w592, error in=w591, "More:Reference Clock:Source"=w589, "More:Synchronization Pulse:Source"=w590) -> (reference out=w594:refnum<k21>, error out=w593:errorcluster)
            }
          }
          n177 = case shown="4, Default" w510 {
            tunnel: w544 -> [w608 w618 w624 _]
            tunnel: w543 -> [w607 w617 w623 _]
            tunnel: [w606 w616 w622 _] -> w542
            tunnel: [w605 w615 w621 _] -> w541
            tunnel: [w604 w614 _ _] -> w540
            tunnel: [w603 w613 _ _] -> w539
            tunnel: w538 -> [w602 w612 _ _]
            tunnel: w537 -> [w601 w611 _ _]
            tunnel: w536 -> [w600 _ _ _]
            tunnel: w535 -> [w599 _ _ _]
            tunnel: [w598 _ _ _] -> w534
            tunnel: [w597 _ _ _] -> w533
            tunnel: w514 -> [w596 w610 w620 _]
            tunnel: w512 -> [w595 w609 w619 _]
            frame 4, Default {
              n178 = property class="DAQmx Timing"(reference=w608, error in=w607, "More:Reference Clock:Source"=w595, "More:Synchronization Pulse:Source"=w596) -> (reference out=w606:refnum<k21>, error out=w605:errorcluster)
              n179 = property class="DAQmx Timing"(reference=w601, error in=w602, "More:Reference Clock:Source"=w595, "More:Synchronization Pulse:Source"=w596) -> (reference out=w603:refnum<k21>, error out=w604:errorcluster)
              n180 = property class="DAQmx Timing"(reference=w600, error in=w599, "More:Reference Clock:Source"=w595, "More:Synchronization Pulse:Source"=w596) -> (reference out=w598:refnum<k21>, error out=w597:errorcluster)
            }
            frame 3 {
              n181 = property class="DAQmx Timing"(reference=w618, error in=w617, "More:Reference Clock:Source"=w609, "More:Synchronization Pulse:Source"=w610) -> (reference out=w616:refnum<k21>, error out=w615:errorcluster)
              n182 = property class="DAQmx Timing"(reference=w611, error in=w612, "More:Reference Clock:Source"=w609, "More:Synchronization Pulse:Source"=w610) -> (reference out=w613:refnum<k21>, error out=w614:errorcluster)
            }
            frame 2 {
              n183 = property class="DAQmx Timing"(reference=w624, error in=w623, "More:Reference Clock:Source"=w619, "More:Synchronization Pulse:Source"=w620) -> (reference out=w622:refnum<k21>, error out=w621:errorcluster)
            }
            frame 1 {
            }
          }
        }
        frame "USB-4431" {
          n184 = call "Get Dev Product Type.vi"("error in (no error)"=w631, "Refnum in"=w635) -> ("error out"=w627:errorcluster, "ProductType"=w632:string, "ActiveDev"=w633:tag, "Refnum out"=w634:refnum<k21>)  [unwired: 6 in]
          n185 = call "44xx_RefClk.vi"("error in (no error)"=w627, "ProductType"=w632, "ActiveDev"=w633, "Refnum in"=w634) -> ("error out"=w628:errorcluster, "RefClk.Src"=w629:tag, "Refnum out"=w630:refnum<k21>)  [unwired: 5 in]
          n186 = property class="DAQmx Timing"(reference=w630, error in=w628, "More:Reference Clock:Source"=w629) -> (reference out=w625:refnum<k21>, error out=w626:errorcluster)
        }
      }
      n187 = call "Get Terminal Name with Device Prefix.vi"("error in (no error)"=w34, "Local Terminal Name"="ai/StartTrigger", "task/channels in"=w33) -> ("error out"=w36:errorcluster, "Terminal Name with Device Prefix"=w60:tag, "task out"=w35:refnum<k21>)  [unwired: 6 in]
      n188 = case shown="1" w30 {
        tunnel: w50 -> [w455 w468 w477 w482]
        tunnel: w51 -> [w454 w467 w476 w481]
        tunnel: [w453 w466 w475 w480] -> w52
        tunnel: [w452 w465 w474 w479] -> w53
        tunnel: w54 -> [w451 w464 w473 _]
        tunnel: w55 -> [w450 w463 w472 _]
        tunnel: w56 -> [w449 w462 _ _]
        tunnel: w57 -> [w448 w461 _ _]
        tunnel: w58 -> [w447 _ _ _]
        tunnel: w59 -> [w446 _ _ _]
        tunnel: w60 -> [w445 w460 w471 w478]
        tunnel: [w444 w459 w470 _] -> w128
        tunnel: [w443 w458 w469 _] -> w129
        tunnel: [w442 w457 _ _] -> w130
        tunnel: [w441 w456 _ _] -> w131
        tunnel: [w440 _ _ _] -> w132
        tunnel: [w439 _ _ _] -> w133
        frame 4, Default {
          n189 = call-poly <vilib>:"DAQmx Trigger.vi"("task/channels in"=w455, "source"=w445, "error in"=w454) -> ("task out"=w453:refnum<k21>, "error out"=w452:errorcluster)  [unwired: 11 in]
          n190 = call-poly <vilib>:"DAQmx Trigger.vi"("task/channels in"=w450, "source"=w445, "error in"=w451) -> ("task out"=w443:refnum<k21>, "error out"=w444:errorcluster)  [unwired: 11 in]
          n191 = call-poly <vilib>:"DAQmx Trigger.vi"("task/channels in"=w449, "source"=w445, "error in"=w448) -> ("task out"=w442:refnum<k21>, "error out"=w441:errorcluster)  [unwired: 11 in]
          n192 = call-poly <vilib>:"DAQmx Trigger.vi"("task/channels in"=w446, "source"=w445, "error in"=w447) -> ("task out"=w439:refnum<k21>, "error out"=w440:errorcluster)  [unwired: 11 in]
        }
        frame 3 {
          n193 = call-poly <vilib>:"DAQmx Trigger.vi"("task/channels in"=w468, "source"=w460, "error in"=w467) -> ("task out"=w466:refnum<k21>, "error out"=w465:errorcluster)  [unwired: 11 in]
          n194 = call-poly <vilib>:"DAQmx Trigger.vi"("task/channels in"=w463, "source"=w460, "error in"=w464) -> ("task out"=w458:refnum<k21>, "error out"=w459:errorcluster)  [unwired: 11 in]
          n195 = call-poly <vilib>:"DAQmx Trigger.vi"("task/channels in"=w462, "source"=w460, "error in"=w461) -> ("task out"=w457:refnum<k21>, "error out"=w456:errorcluster)  [unwired: 11 in]
        }
        frame 2 {
          n196 = call-poly <vilib>:"DAQmx Trigger.vi"("task/channels in"=w477, "source"=w471, "error in"=w476) -> ("task out"=w475:refnum<k21>, "error out"=w474:errorcluster)  [unwired: 11 in]
          n197 = call-poly <vilib>:"DAQmx Trigger.vi"("task/channels in"=w472, "source"=w471, "error in"=w473) -> ("task out"=w469:refnum<k21>, "error out"=w470:errorcluster)  [unwired: 11 in]
        }
        frame 1 {
          n198 = call-poly <vilib>:"DAQmx Trigger.vi"("task/channels in"=w482, "source"=w478, "error in"=w481) -> ("task out"=w480:refnum<k21>, "error out"=w479:errorcluster)  [unwired: 11 in]
        }
      }
      n199 = case shown="2" w157 {
        tunnel: w39 -> [w495 w504 w509 _]
        tunnel: w40 -> [w494 w503 w508 _]
        tunnel: w41 -> [w493 w502 _ _]
        tunnel: w42 -> [w492 w501 _ _]
        tunnel: w47 -> [w491 _ _ _]
        tunnel: w48 -> [w490 _ _ _]
        tunnel: w60 -> [w489 w500 w507 _]
        tunnel: [w488 _ _ _] -> w122
        tunnel: [w487 w499 _ _] -> w123
        tunnel: [w486 w498 w506 _] -> w124
        tunnel: [w485 w497 w505 _] -> w125
        tunnel: [w484 w496 _ _] -> w126
        tunnel: [w483 _ _ _] -> w127
        frame 4, Default {
          n200 = call-poly <vilib>:"DAQmx Trigger.vi"("task/channels in"=w495, "source"=w489, "error in"=w494) -> ("task out"=w486:refnum<k21>, "error out"=w485:errorcluster)  [unwired: 11 in]
          n201 = call-poly <vilib>:"DAQmx Trigger.vi"("task/channels in"=w492, "source"=w489, "error in"=w493) -> ("task out"=w487:refnum<k21>, "error out"=w484:errorcluster)  [unwired: 11 in]
          n202 = call-poly <vilib>:"DAQmx Trigger.vi"("task/channels in"=w491, "source"=w489, "error in"=w490) -> ("task out"=w488:refnum<k21>, "error out"=w483:errorcluster)  [unwired: 11 in]
        }
        frame 3 {
          n203 = call-poly <vilib>:"DAQmx Trigger.vi"("task/channels in"=w504, "source"=w500, "error in"=w503) -> ("task out"=w498:refnum<k21>, "error out"=w497:errorcluster)  [unwired: 11 in]
          n204 = call-poly <vilib>:"DAQmx Trigger.vi"("task/channels in"=w501, "source"=w500, "error in"=w502) -> ("task out"=w499:refnum<k21>, "error out"=w496:errorcluster)  [unwired: 11 in]
        }
        frame 2 {
          n205 = call-poly <vilib>:"DAQmx Trigger.vi"("task/channels in"=w509, "source"=w507, "error in"=w508) -> ("task out"=w506:refnum<k21>, "error out"=w505:errorcluster)  [unwired: 11 in]
        }
        frame 1 {
        }
      }
      n206 = case shown="\"USB-4431\"" w155 {
        tunnel: w35 -> [w342 w438]
        tunnel: w36 -> [w341 w437]
        tunnel: [w340 w437] -> w141
        tunnel: [w339 w438] -> w140
        tunnel: [w338 w436] -> w49
        tunnel: w52 -> [w337 w430]
        tunnel: w53 -> [w336 w429]
        tunnel: [w335 w434] -> w61
        tunnel: [w334 w432] -> w62
        tunnel: [w333 w435] -> w63
        tunnel: [w332 w433] -> w64
        tunnel: [w331 w431] -> w65
        tunnel: [w330 w430] -> w66
        tunnel: [w329 w428] -> w67
        tunnel: [w328 w426] -> w68
        tunnel: [w327 w429] -> w69
        tunnel: [w326 w427] -> w70
        tunnel: [w325 w425] -> w71
        tunnel: [w324 w424] -> w72
        tunnel: [w323 w423] -> w73
        tunnel: w122 -> [w322 w432]
        tunnel: w123 -> [w321 w434]
        tunnel: w124 -> [w320 w436]
        tunnel: w125 -> [w319 w435]
        tunnel: w126 -> [w318 w433]
        tunnel: w127 -> [w317 w431]
        tunnel: w128 -> [w316 w427]
        tunnel: w129 -> [w315 w428]
        tunnel: w130 -> [w314 w426]
        tunnel: w131 -> [w313 w425]
        tunnel: w132 -> [w312 w423]
        tunnel: w133 -> [w311 w424]
        tunnel: w30 -> [w298 _]
        tunnel: w157 -> [w297 _]
        frame Default {
          n207 = case shown="4, Default" w297 {
            tunnel: [w407 w417 w422 _] -> w338
            tunnel: [w406 w416 _ _] -> w335
            tunnel: [w405 _ _ _] -> w334
            tunnel: [w404 w415 w421 _] -> w333
            tunnel: [w403 w414 _ _] -> w332
            tunnel: [w402 _ _ _] -> w331
            tunnel: w322 -> [w401 _ _ _]
            tunnel: w321 -> [w400 w413 _ _]
            tunnel: w320 -> [w399 w412 w420 _]
            tunnel: w319 -> [w398 w411 w419 _]
            tunnel: w318 -> [w397 w410 _ _]
            tunnel: w317 -> [w396 _ _ _]
            tunnel: [w395 w409 w418 _] -> w305
            tunnel: [w394 w408 _ _] -> w304
            tunnel: [w393 _ _ _] -> w303
            frame 4, Default {
              n208 = property class="DAQmx Timing"(reference=w399, error in=w398) -> (reference out=w407:refnum<k21>, error out=w404:errorcluster, "SyncPulse.SyncTime"=w395:dbl)
              n209 = property class="DAQmx Timing"(reference=w400, error in=w397) -> (reference out=w406:refnum<k21>, error out=w403:errorcluster, "SyncPulse.SyncTime"=w394:dbl)
              n210 = property class="DAQmx Timing"(reference=w401, error in=w396) -> (reference out=w405:refnum<k21>, error out=w402:errorcluster, "SyncPulse.SyncTime"=w393:dbl)
            }
            frame 3 {
              n211 = property class="DAQmx Timing"(reference=w412, error in=w411) -> (reference out=w417:refnum<k21>, error out=w415:errorcluster, "SyncPulse.SyncTime"=w409:dbl)
              n212 = property class="DAQmx Timing"(reference=w413, error in=w410) -> (reference out=w416:refnum<k21>, error out=w414:errorcluster, "SyncPulse.SyncTime"=w408:dbl)
            }
            frame 2 {
              n213 = property class="DAQmx Timing"(reference=w420, error in=w419) -> (reference out=w422:refnum<k21>, error out=w421:errorcluster, "SyncPulse.SyncTime"=w418:dbl)
            }
            frame 1 {
            }
          }
          n214 = case shown="2" w298 {
            tunnel: w337 -> [w362 w377 w387 w392]
            tunnel: w336 -> [w361 w376 w386 w391]
            tunnel: [w360 w375 w385 w390] -> w330
            tunnel: [w359 w374 w384 _] -> w329
            tunnel: [w358 w373 _ _] -> w328
            tunnel: [w357 w372 w383 w389] -> w327
            tunnel: [w356 w371 w382 _] -> w326
            tunnel: [w355 w370 _ _] -> w325
            tunnel: [w354 _ _ _] -> w324
            tunnel: [w353 _ _ _] -> w323
            tunnel: w316 -> [w352 w369 w381 _]
            tunnel: w315 -> [w351 w368 w380 _]
            tunnel: w314 -> [w350 w367 _ _]
            tunnel: w313 -> [w349 w366 _ _]
            tunnel: w312 -> [w348 _ _ _]
            tunnel: w311 -> [w347 _ _ _]
            tunnel: [w346 w365 w379 w388] -> w302
            tunnel: [w345 w364 w378 _] -> w301
            tunnel: [w344 w363 _ _] -> w300
            tunnel: [w343 _ _ _] -> w299
            frame 4, Default {
              n215 = property class="DAQmx Timing"(reference=w362, error in=w361) -> (reference out=w360:refnum<k21>, error out=w357:errorcluster, "SyncPulse.SyncTime"=w346:dbl)
              n216 = property class="DAQmx Timing"(reference=w351, error in=w352) -> (reference out=w359:refnum<k21>, error out=w356:errorcluster, "SyncPulse.SyncTime"=w345:dbl)
              n217 = property class="DAQmx Timing"(reference=w350, error in=w349) -> (reference out=w358:refnum<k21>, error out=w355:errorcluster, "SyncPulse.SyncTime"=w344:dbl)
              n218 = property class="DAQmx Timing"(reference=w347, error in=w348) -> (reference out=w354:refnum<k21>, error out=w353:errorcluster, "SyncPulse.SyncTime"=w343:dbl)
            }
            frame 3 {
              n219 = property class="DAQmx Timing"(reference=w377, error in=w376) -> (reference out=w375:refnum<k21>, error out=w372:errorcluster, "SyncPulse.SyncTime"=w365:dbl)
              n220 = property class="DAQmx Timing"(reference=w368, error in=w369) -> (reference out=w374:refnum<k21>, error out=w371:errorcluster, "SyncPulse.SyncTime"=w364:dbl)
              n221 = property class="DAQmx Timing"(reference=w367, error in=w366) -> (reference out=w373:refnum<k21>, error out=w370:errorcluster, "SyncPulse.SyncTime"=w363:dbl)
            }
            frame 2 {
              n222 = property class="DAQmx Timing"(reference=w387, error in=w386) -> (reference out=w385:refnum<k21>, error out=w383:errorcluster, "SyncPulse.SyncTime"=w379:dbl)
              n223 = property class="DAQmx Timing"(reference=w380, error in=w381) -> (reference out=w384:refnum<k21>, error out=w382:errorcluster, "SyncPulse.SyncTime"=w378:dbl)
            }
            frame 1 {
              n224 = property class="DAQmx Timing"(reference=w392, error in=w391) -> (reference out=w390:refnum<k21>, error out=w389:errorcluster, "SyncPulse.SyncTime"=w388:dbl)
            }
          }
          n225 = property class="DAQmx Timing"(reference=w342, error in=w341) -> (reference out=w308:refnum<k21>, error out=w309:errorcluster, "SyncPulse.SyncTime"=w310:dbl)
          n226 = Build Array(w310, w305, w304, w303, w302, w301, w300, w299) -> (w307:dbl[])
          n227 = Array Max & Min(array=w307) -> (max value=w306:dbl)  [unwired: 3 out]
          n228 = property class="DAQmx Timing"(reference=w308, error in=w309, "SyncPulse.MinDelayToStart"=w306) -> (reference out=w339:refnum<k21>, error out=w340:errorcluster)
        }
        frame "USB-4431" {
        }
      }
      n229 = Not(x=w28) -> (.not. x?=w29:bool)
      n230 = call "4461 - Create AO waveforms.vi"("sampling info"=w12, "error in (no error)"=w20, "reset signal"=w29, "AO"=w9) -> ("error out"=w138:errorcluster, "AO Array"=w142:waveform(dbl)[])  [unwired: 4 in, 2 out]
      n231 = call "4461 - Create Reference Waveforms.vi"("sampling info"=w12, "reset signal"=w29, "Lockin"=w8) -> ()  [unwired: 5 in, 4 out]
      n232 = case shown="\"USB-4431\"" w155 {
        tunnel: [w203 w209] -> w78
        tunnel: [w202 w208] -> w79
        tunnel: [w201 w207] -> w80
        tunnel: [w199 w205] -> w139
        tunnel: w142 -> [w198 w204]
        frame "USB-4431" {
          n233 = Index Array(array=w198) -> (element #1=w200:waveform(dbl), element #2=w197:waveform(dbl), element #3=w196:waveform(dbl), element #4=w195:waveform(dbl))  [unwired: 4 in]
          n234 = Build Array(w200) -> (w199:waveform(dbl)[])
          n235 = Build Array(w197) -> (w203:waveform(dbl)[])
          n236 = Build Array(w196) -> (w202:waveform(dbl)[])
          n237 = Build Array(w195) -> (w201:waveform(dbl)[])
        }
        frame Default {
          n238 = Index Array(array=w204) -> (element #1=w206:waveform(dbl), element #2=w216:waveform(dbl), element #3=w215:waveform(dbl), element #4=w214:waveform(dbl), element #5=w213:waveform(dbl), element #6=w212:waveform(dbl), element #7=w211:waveform(dbl), element #8=w210:waveform(dbl))  [unwired: 8 in]
          n239 = Build Array(w206, w216) -> (w205:waveform(dbl)[])
          n240 = Build Array(w215, w214) -> (w209:waveform(dbl)[])
          n241 = Build Array(w213, w212) -> (w208:waveform(dbl)[])
          n242 = Build Array(w211, w210) -> (w207:waveform(dbl)[])
        }
      }
      n243 = flat-sequence {
        tunnel: w141 -> [w1137]
        tunnel: w140 -> [w1136]
        tunnel: [w1137] -> w194
        tunnel: [w1159] -> w193
        tunnel: w49 -> [w1159]
        tunnel: [w1158] -> w192
        tunnel: w61 -> [w1158]
        tunnel: [w1157] -> w191
        tunnel: w62 -> [w1157]
        tunnel: [w1156] -> w190
        tunnel: w63 -> [w1156]
        tunnel: [w1155] -> w189
        tunnel: w64 -> [w1155]
        tunnel: [w1154] -> w188
        tunnel: w65 -> [w1154]
        tunnel: w66 -> [w1134]
        tunnel: [w1143] -> w187
        tunnel: w67 -> [w1144]
        tunnel: [w1147] -> w186
        tunnel: w68 -> [w1146]
        tunnel: [w1135] -> w185
        tunnel: w69 -> [w1135]
        tunnel: w70 -> [w1145]
        tunnel: [w1148] -> w184
        tunnel: w71 -> [w1149]
        tunnel: [w1150] -> w183
        tunnel: w72 -> [w1153]
        tunnel: [w1151] -> w182
        tunnel: w73 -> [w1152]
        tunnel: [w1142] -> w181
        tunnel: w78 -> [w1141]
        tunnel: w79 -> [w1140]
        tunnel: w80 -> [w1139]
        tunnel: w30 -> [w1138]
        tunnel: w139 -> [w1133]
        tunnel: [w1136] -> w180
        tunnel: [w1134] -> w179
        tunnel: [w1133] -> w178
        tunnel: [w1208] -> w177
        tunnel: [w1207] -> w176
        tunnel: w194 -> [w1207]
        tunnel: [w1206] -> w175
        tunnel: w193 -> [w1206]
        tunnel: [w1205] -> w174
        tunnel: w192 -> [w1205]
        tunnel: [w1204] -> w173
        tunnel: w191 -> [w1204]
        tunnel: [w1203] -> w172
        tunnel: w190 -> [w1203]
        tunnel: [w1202] -> w171
        tunnel: w189 -> [w1202]
        tunnel: [w1201] -> w170
        tunnel: w188 -> [w1201]
        tunnel: [w1193] -> w169
        tunnel: [w1200] -> w168
        tunnel: w187 -> [w1200]
        tunnel: [w1199] -> w167
        tunnel: w186 -> [w1199]
        tunnel: [w1192] -> w166
        tunnel: w185 -> [w1191]
        tunnel: [w1198] -> w165
        tunnel: [w1197] -> w164
        tunnel: w184 -> [w1197]
        tunnel: [w1196] -> w163
        tunnel: w183 -> [w1196]
        tunnel: [w1195] -> w162
        tunnel: w182 -> [w1195]
        tunnel: w181 -> [w1198]
        tunnel: w180 -> [w1208]
        tunnel: w179 -> [w1194]
        tunnel: w178 -> [w1190]
        tunnel: [w1240] -> w31
        tunnel: [w1239] -> w32
        tunnel: w177 -> [w1240]
        tunnel: w176 -> [w1239]
        tunnel: w175 -> [w1238]
        tunnel: w174 -> [w1237]
        tunnel: w173 -> [w1236]
        tunnel: w172 -> [w1235]
        tunnel: w171 -> [w1234]
        tunnel: w170 -> [w1233]
        tunnel: w169 -> [w1232]
        tunnel: w168 -> [w1231]
        tunnel: w167 -> [w1230]
        tunnel: w166 -> [w1229]
        tunnel: w165 -> [w1228]
        tunnel: w164 -> [w1227]
        tunnel: w163 -> [w1226]
        tunnel: w162 -> [w1225]
        tunnel: [w1224] -> w102
        tunnel: [w1223] -> w103
        tunnel: [w1222] -> w104
        tunnel: [w1221] -> w74
        tunnel: [w1220] -> w75
        tunnel: [w1219] -> w76
        tunnel: [w1218] -> w119
        tunnel: [w1217] -> w107
        tunnel: [w1216] -> w106
        tunnel: [w1215] -> w105
        tunnel: [w1214] -> w115
        tunnel: [w1213] -> w81
        tunnel: [w1212] -> w82
        tunnel: [w1211] -> w83
        tunnel: w157 -> [w1210]
        tunnel: w30 -> [w1209]
        frame #0 {
          n244 = case shown="1" w1138 {
            tunnel: w1153 -> [w1174 _ _ _]
            tunnel: w1152 -> [w1173 _ _ _]
            tunnel: [w1172 _ _ _] -> w1151
            tunnel: [w1171 _ _ _] -> w1150
            tunnel: w1149 -> [w1170 w1184 _ _]
            tunnel: [w1169 w1183 _ _] -> w1148
            tunnel: [w1168 w1182 _ _] -> w1147
            tunnel: w1146 -> [w1167 w1181 _ _]
            tunnel: w1145 -> [w1166 w1180 w1189 _]
            tunnel: w1144 -> [w1165 w1179 w1188 _]
            tunnel: [w1164 w1178 w1187 _] -> w1143
            tunnel: [w1163 w1177 w1186 _] -> w1142
            tunnel: w1141 -> [w1162 w1176 w1185 _]
            tunnel: w1140 -> [w1161 w1175 _ _]
            tunnel: w1139 -> [w1160 _ _ _]
            frame 4, Default {
              n245 = call-poly <vilib>:"DAQmx Write.vi"("task/channels in"=w1167, "data"=w1161, "error in"=w1170) -> ("task out"=w1168:refnum<k21>, "error out"=w1169:errorcluster)  [unwired: 10 in, 1 out]
              n246 = call-poly <vilib>:"DAQmx Write.vi"("task/channels in"=w1174, "data"=w1160, "error in"=w1173) -> ("task out"=w1171:refnum<k21>, "error out"=w1172:errorcluster)  [unwired: 10 in, 1 out]
              n247 = call-poly <vilib>:"DAQmx Write.vi"("task/channels in"=w1165, "data"=w1162, "error in"=w1166) -> ("task out"=w1164:refnum<k21>, "error out"=w1163:errorcluster)  [unwired: 10 in, 1 out]
            }
            frame 3 {
              n248 = call-poly <vilib>:"DAQmx Write.vi"("task/channels in"=w1181, "data"=w1175, "error in"=w1184) -> ("task out"=w1182:refnum<k21>, "error out"=w1183:errorcluster)  [unwired: 10 in, 1 out]
              n249 = call-poly <vilib>:"DAQmx Write.vi"("task/channels in"=w1179, "data"=w1176, "error in"=w1180) -> ("task out"=w1178:refnum<k21>, "error out"=w1177:errorcluster)  [unwired: 10 in, 1 out]
            }
            frame 2 {
              n250 = call-poly <vilib>:"DAQmx Write.vi"("task/channels in"=w1188, "data"=w1185, "error in"=w1189) -> ("task out"=w1187:refnum<k21>, "error out"=w1186:errorcluster)  [unwired: 10 in, 1 out]
            }
            frame 1 {
            }
          }
        }
        frame #1 {
          n251 = call-poly <vilib>:"DAQmx Write.vi"("task/channels in"=w1194, "data"=w1190, "error in"=w1191) -> ("task out"=w1193:refnum<k21>, "error out"=w1192:errorcluster)  [unwired: 10 in, 1 out]
        }
        frame #2 {
          n252 = case shown="3" w1210 {
            tunnel: w1238 -> [w1292 w1300 w1304 _]
            tunnel: w1237 -> [w1291 w1299 _ _]
            tunnel: w1236 -> [w1290 _ _ _]
            tunnel: w1235 -> [w1289 w1298 w1303 _]
            tunnel: w1234 -> [w1288 w1297 _ _]
            tunnel: w1233 -> [w1287 _ _ _]
            tunnel: [w1286 w1296 w1302 _] -> w1224
            tunnel: [w1285 w1295 _ _] -> w1223
            tunnel: [w1284 _ _ _] -> w1222
            tunnel: [w1283 w1294 w1301 _] -> w1217
            tunnel: [w1282 w1293 _ _] -> w1216
            tunnel: [w1281 _ _ _] -> w1215
            frame 4, Default {
              n253 = call <vilib>:"DAQmx Start Task.vi"("task/channels in"=w1292, "error in"=w1289) -> ("task out"=w1286:refnum<k21>, "error out"=w1283:errorcluster)  [unwired: 12 in]
              n254 = call <vilib>:"DAQmx Start Task.vi"("task/channels in"=w1291, "error in"=w1288) -> ("task out"=w1285:refnum<k21>, "error out"=w1282:errorcluster)  [unwired: 12 in]
              n255 = call <vilib>:"DAQmx Start Task.vi"("task/channels in"=w1290, "error in"=w1287) -> ("task out"=w1284:refnum<k21>, "error out"=w1281:errorcluster)  [unwired: 12 in]
            }
            frame 3 {
              n256 = call <vilib>:"DAQmx Start Task.vi"("task/channels in"=w1300, "error in"=w1298) -> ("task out"=w1296:refnum<k21>, "error out"=w1294:errorcluster)  [unwired: 12 in]
              n257 = call <vilib>:"DAQmx Start Task.vi"("task/channels in"=w1299, "error in"=w1297) -> ("task out"=w1295:refnum<k21>, "error out"=w1293:errorcluster)  [unwired: 12 in]
            }
            frame 2 {
              n258 = call <vilib>:"DAQmx Start Task.vi"("task/channels in"=w1304, "error in"=w1303) -> ("task out"=w1302:refnum<k21>, "error out"=w1301:errorcluster)  [unwired: 12 in]
            }
            frame 1 {
            }
          }
          n259 = case shown="1" w1209 {
            tunnel: w1232 -> [w1256 w1268 w1276 w1280]
            tunnel: w1231 -> [w1255 w1267 w1275 _]
            tunnel: w1230 -> [w1254 w1266 _ _]
            tunnel: w1229 -> [w1253 w1265 w1274 w1279]
            tunnel: w1228 -> [w1252 w1264 w1273 _]
            tunnel: w1227 -> [w1251 w1263 _ _]
            tunnel: w1226 -> [w1250 _ _ _]
            tunnel: w1225 -> [w1249 _ _ _]
            tunnel: [w1248 w1262 w1272 w1278] -> w1221
            tunnel: [w1247 w1261 w1271 _] -> w1220
            tunnel: [w1246 w1260 _ _] -> w1219
            tunnel: [w1245 _ _ _] -> w1218
            tunnel: [w1244 w1259 w1270 w1277] -> w1214
            tunnel: [w1243 w1258 w1269 _] -> w1213
            tunnel: [w1242 w1257 _ _] -> w1212
            tunnel: [w1241 _ _ _] -> w1211
            frame 4, Default {
              n260 = call <vilib>:"DAQmx Start Task.vi"("task/channels in"=w1256, "error in"=w1253) -> ("task out"=w1248:refnum<k21>, "error out"=w1244:errorcluster)  [unwired: 12 in]
              n261 = call <vilib>:"DAQmx Start Task.vi"("task/channels in"=w1255, "error in"=w1252) -> ("task out"=w1247:refnum<k21>, "error out"=w1243:errorcluster)  [unwired: 12 in]
              n262 = call <vilib>:"DAQmx Start Task.vi"("task/channels in"=w1254, "error in"=w1251) -> ("task out"=w1246:refnum<k21>, "error out"=w1242:errorcluster)  [unwired: 12 in]
              n263 = call <vilib>:"DAQmx Start Task.vi"("task/channels in"=w1250, "error in"=w1249) -> ("task out"=w1245:refnum<k21>, "error out"=w1241:errorcluster)  [unwired: 12 in]
            }
            frame 3 {
              n264 = call <vilib>:"DAQmx Start Task.vi"("task/channels in"=w1268, "error in"=w1265) -> ("task out"=w1262:refnum<k21>, "error out"=w1259:errorcluster)  [unwired: 12 in]
              n265 = call <vilib>:"DAQmx Start Task.vi"("task/channels in"=w1267, "error in"=w1264) -> ("task out"=w1261:refnum<k21>, "error out"=w1258:errorcluster)  [unwired: 12 in]
              n266 = call <vilib>:"DAQmx Start Task.vi"("task/channels in"=w1266, "error in"=w1263) -> ("task out"=w1260:refnum<k21>, "error out"=w1257:errorcluster)  [unwired: 12 in]
            }
            frame 2 {
              n267 = call <vilib>:"DAQmx Start Task.vi"("task/channels in"=w1276, "error in"=w1274) -> ("task out"=w1272:refnum<k21>, "error out"=w1270:errorcluster)  [unwired: 12 in]
              n268 = call <vilib>:"DAQmx Start Task.vi"("task/channels in"=w1275, "error in"=w1273) -> ("task out"=w1271:refnum<k21>, "error out"=w1269:errorcluster)  [unwired: 12 in]
            }
            frame 1 {
              n269 = call <vilib>:"DAQmx Start Task.vi"("task/channels in"=w1280, "error in"=w1279) -> ("task out"=w1278:refnum<k21>, "error out"=w1277:errorcluster)  [unwired: 12 in]
            }
          }
        }
      }
      n270 = call <vilib>:"DAQmx Start Task.vi"("task/channels in"=w31, "error in"=w32) -> ("task out"=w101:refnum<k21>, "error out"=w121:errorcluster)  [unwired: 12 in]
      n271 = while {
        tunnel: w101 -> [w1060]
        tunnel: w121 -> [w1059]
        tunnel: [w1043] -> w114
        tunnel: [w1058] -> w100
        tunnel: w102 -> [w1057]
        tunnel: w103 -> [w1055]
        tunnel: w104 -> [w1056]
        tunnel: w105 -> [w1054]
        tunnel: w106 -> [w1053]
        tunnel: w107 -> [w1052]
        tunnel: w159 -> [w1051]
        tunnel: [w1050] -> w108
        tunnel: [w1044] -> w109
        tunnel: [w1049] -> w110
        tunnel: [w1046] -> w111
        tunnel: [w1048] -> w112
        tunnel: [w1047] -> w113
        tunnel: w157 -> [w1042]
        stop <- w1045 stop-if-true
        n272 = case shown="1" w1042 {
          tunnel: w1060 -> [w1087 w1108 w1123 w1132]
          tunnel: w1059 -> [w1086 w1107 w1122 w1131]
          tunnel: [w1085 w1106 w1121 w1130] -> w1058
          tunnel: w1057 -> [w1084 w1105 w1120 _]
          tunnel: w1056 -> [w1083 _ _ _]
          tunnel: w1055 -> [w1082 w1104 _ _]
          tunnel: w1054 -> [w1081 _ _ _]
          tunnel: w1053 -> [w1080 w1103 _ _]
          tunnel: w1052 -> [w1079 w1102 w1119 _]
          tunnel: w1051 -> [w1078 w1101 w1118 w1129]
          tunnel: [w1073 w1097 w1115 _] -> w1050
          tunnel: [w1072 w1096 _ _] -> w1049
          tunnel: [w1071 _ _ _] -> w1048
          tunnel: [w1070 _ _ _] -> w1047
          tunnel: [w1069 w1095 _ _] -> w1046
          tunnel: [w1068 w1094 w1114 w1127] -> w1045
          tunnel: [w1067 w1093 w1113 _] -> w1044
          tunnel: [w1066 w1092 w1112 w1126] -> w1043
          frame 4, Default {
            n273 = property class="DAQmx Read"(reference=w1087, error in=w1086) -> (reference out=w1085:refnum<k21>, error out=w1066:errorcluster, "AvailSampPerChan"=w1064:u32)
            n274 = property class="DAQmx Read"(reference=w1084, error in=w1079) -> (reference out=w1073:refnum<k21>, error out=w1067:errorcluster, "AvailSampPerChan"=w1063:u32)
            n275 = property class="DAQmx Read"(reference=w1082, error in=w1080) -> (reference out=w1072:refnum<k21>, error out=w1069:errorcluster, "AvailSampPerChan"=w1062:u32)
            n276 = property class="DAQmx Read"(reference=w1083, error in=w1081) -> (reference out=w1071:refnum<k21>, error out=w1070:errorcluster, "AvailSampPerChan"=w1061:u32)
            n277 = Greater Or Equal?(x=w1064, y=w1078) -> (x >= y?=w1077:bool)
            n278 = Greater Or Equal?(x=w1063, y=w1078) -> (x >= y?=w1076:bool)
            n279 = Greater Or Equal?(x=w1062, y=w1078) -> (x >= y?=w1075:bool)
            n280 = Greater Or Equal?(x=w1061, y=w1078) -> (x >= y?=w1074:bool)
            n281 = Compound Arithmetic op=AND(w1077, w1076, w1075, w1074) -> (w1065:bool)
            n282 = Compound Arithmetic op=OR(w1066, w1067, w1069, w1070, w1065) -> (w1068:bool)
          }
          frame 3 {
            n283 = property class="DAQmx Read"(reference=w1108, error in=w1107) -> (reference out=w1106:refnum<k21>, error out=w1092:errorcluster, "AvailSampPerChan"=w1090:u32)
            n284 = property class="DAQmx Read"(reference=w1105, error in=w1102) -> (reference out=w1097:refnum<k21>, error out=w1093:errorcluster, "AvailSampPerChan"=w1089:u32)
            n285 = property class="DAQmx Read"(reference=w1104, error in=w1103) -> (reference out=w1096:refnum<k21>, error out=w1095:errorcluster, "AvailSampPerChan"=w1088:u32)
            n286 = Greater Or Equal?(x=w1090, y=w1101) -> (x >= y?=w1100:bool)
            n287 = Greater Or Equal?(x=w1089, y=w1101) -> (x >= y?=w1099:bool)
            n288 = Greater Or Equal?(x=w1088, y=w1101) -> (x >= y?=w1098:bool)
            n289 = Compound Arithmetic op=AND(w1100, w1099, w1098) -> (w1091:bool)
            n290 = Compound Arithmetic op=OR(w1092, w1093, w1095, w1091) -> (w1094:bool)
          }
          frame 2 {
            n291 = property class="DAQmx Read"(reference=w1123, error in=w1122) -> (reference out=w1121:refnum<k21>, error out=w1112:errorcluster, "AvailSampPerChan"=w1110:u32)
            n292 = property class="DAQmx Read"(reference=w1120, error in=w1119) -> (reference out=w1115:refnum<k21>, error out=w1113:errorcluster, "AvailSampPerChan"=w1109:u32)
            n293 = Greater Or Equal?(x=w1110, y=w1118) -> (x >= y?=w1117:bool)
            n294 = Greater Or Equal?(x=w1109, y=w1118) -> (x >= y?=w1116:bool)
            n295 = Compound Arithmetic op=AND(w1117, w1116) -> (w1111:bool)
            n296 = Compound Arithmetic op=OR(w1112, w1113, w1111) -> (w1114:bool)
          }
          frame 1 {
            n297 = property class="DAQmx Read"(reference=w1132, error in=w1131) -> (reference out=w1130:refnum<k21>, error out=w1126:errorcluster, "AvailSampPerChan"=w1124:u32)
            n298 = Greater Or Equal?(x=w1124, y=w1129) -> (x >= y?=w1128:bool)
            n299 = Compound Arithmetic op=AND(w1128) -> (w1125:bool)
            n300 = Compound Arithmetic op=OR(w1126, w1125) -> (w1127:bool)
          }
        }
      }
      n301 = case shown="3" w157 {
        tunnel: [w263 w278 w289 w296] -> w17
        tunnel: w100 -> [w262 w277 w288 w295]
        tunnel: w108 -> [w261 w276 w287 _]
        tunnel: w109 -> [w260 w275 w286 _]
        tunnel: w110 -> [w259 w274 _ _]
        tunnel: w111 -> [w258 w273 _ _]
        tunnel: w112 -> [w257 _ _ _]
        tunnel: w113 -> [w256 _ _ _]
        tunnel: w114 -> [w255 w272 w285 w294]
        tunnel: w159 -> [w247 w266 w281 w292]
        tunnel: [w245 w264 w279 w290] -> w137
        frame 4, Default {
          n302 = call-poly <vilib>:"DAQmx Read.vi"("task/channels in"=w262, "number of samples per channel"=w247, "error in"=w255) -> ("task out"=w254:refnum<k21>, "error out"=w246:errorcluster)  [unwired: 10 in, 1 out]
          n303 = call-poly <vilib>:"DAQmx Read.vi"("task/channels in"=w261, "number of samples per channel"=w247, "error in"=w260) -> ("task out"=w253:refnum<k21>, "error out"=w252:errorcluster)  [unwired: 10 in, 1 out]
          n304 = call-poly <vilib>:"DAQmx Read.vi"("task/channels in"=w259, "number of samples per channel"=w247, "error in"=w258) -> ("task out"=w248:refnum<k21>, "error out"=w251:errorcluster)  [unwired: 10 in, 1 out]
          n305 = call-poly <vilib>:"DAQmx Read.vi"("task/channels in"=w257, "number of samples per channel"=w247, "error in"=w256) -> ("task out"=w249:refnum<k21>, "error out"=w250:errorcluster)  [unwired: 10 in, 1 out]
          n306 = Build Array(w254, w253, w248, w249) -> (w263:refnum<k21>[])
          n307 = Merge Errors(w246, w252, w251, w250) -> (w245:errorcluster)
        }
        frame 3 {
          n308 = call-poly <vilib>:"DAQmx Read.vi"("task/channels in"=w277, "number of samples per channel"=w266, "error in"=w272) -> ("task out"=w271:refnum<k21>, "error out"=w265:errorcluster)  [unwired: 10 in, 1 out]
          n309 = call-poly <vilib>:"DAQmx Read.vi"("task/channels in"=w276, "number of samples per channel"=w266, "error in"=w275) -> ("task out"=w270:refnum<k21>, "error out"=w269:errorcluster)  [unwired: 10 in, 1 out]
          n310 = call-poly <vilib>:"DAQmx Read.vi"("task/channels in"=w274, "number of samples per channel"=w266, "error in"=w273) -> ("task out"=w267:refnum<k21>, "error out"=w268:errorcluster)  [unwired: 10 in, 1 out]
          n311 = Build Array(w271, w270, w267) -> (w278:refnum<k21>[])
          n312 = Merge Errors(w265, w269, w268) -> (w264:errorcluster)
        }
        frame 2 {
          n313 = call-poly <vilib>:"DAQmx Read.vi"("task/channels in"=w288, "number of samples per channel"=w281, "error in"=w285) -> ("task out"=w284:refnum<k21>, "error out"=w280:errorcluster)  [unwired: 10 in, 1 out]
          n314 = call-poly <vilib>:"DAQmx Read.vi"("task/channels in"=w287, "number of samples per channel"=w281, "error in"=w286) -> ("task out"=w283:refnum<k21>, "error out"=w282:errorcluster)  [unwired: 10 in, 1 out]
          n315 = Build Array(w284, w283) -> (w289:refnum<k21>[])
          n316 = Merge Errors(w280, w282) -> (w279:errorcluster)
        }
        frame 1 {
          n317 = call-poly <vilib>:"DAQmx Read.vi"("task/channels in"=w295, "number of samples per channel"=w292, "error in"=w294) -> ("task out"=w293:refnum<k21>, "error out"=w291:errorcluster)  [unwired: 10 in, 1 out]
          n318 = Build Array(w293) -> (w296:refnum<k21>[])
          n319 = Merge Errors(w291) -> (w290:errorcluster)
        }
      }
      n320 = case shown="4, Default" w30 {
        tunnel: w74 -> [w226 w234 w240 w244]
        tunnel: w75 -> [w225 w233 w239 _]
        tunnel: w76 -> [w224 w232 _ _]
        tunnel: [w223 w231 w238 w243] -> w16
        tunnel: w81 -> [w222 w230 w237 _]
        tunnel: w82 -> [w221 w229 _ _]
        tunnel: w83 -> [w220 _ _ _]
        tunnel: w115 -> [w219 w228 w236 w242]
        tunnel: [w218 w227 w235 w241] -> w118
        tunnel: w119 -> [w217 _ _ _]
        frame 4, Default {
          n321 = Build Array(w226, w225, w224, w217) -> (w223:refnum<k21>[])
          n322 = Merge Errors(w219, w222, w221, w220) -> (w218:errorcluster)
        }
        frame 3 {
          n323 = Build Array(w234, w233, w232) -> (w231:refnum<k21>[])
          n324 = Merge Errors(w228, w230, w229) -> (w227:errorcluster)
        }
        frame 2 {
          n325 = Build Array(w240, w239) -> (w238:refnum<k21>[])
          n326 = Merge Errors(w236, w237) -> (w235:errorcluster)
        }
        frame 1 {
          n327 = Build Array(w244) -> (w243:refnum<k21>[])
          n328 = Merge Errors(w242) -> (w241:errorcluster)
        }
      }
      n329 = Merge Errors(w137, w118, w138) -> (w21:errorcluster)
      n330 = Bundle By Name(cluster=w19, "AI task"=w17, "AO Task"=w16, "sampling info"=w12, "sample mode"=w11) -> (w18:refnum<class "LockinDAQ.lvclass">)
    }
    frame Error {
    }
  }
  "error out" <- w4
  "LockinDAQ out" <- w2
